vi "UHR-Fleezers Control (fpga) - 11.5.vi"() -> ()   [LabVIEW 2012]
doc: "UHR-Fleezers Instrument Control Code (fpga)"
uses:
  <vilib>/Platform/TimedLoop/XDataNode/timing_clust.ctl
  <vilib>/Platform/TimedLoop/XDataNode/nitl_modes.ctl
  <vilib>/Platform/TimedLoop/XDataNode/wakeup.ctl
  <vilib>/rvi/eio/common/nirviEmuTemplateMethod_errors.vi
  <vilib>/rvi/Emulation/niFpgaSctlEmulationGetInTimedLoop.vi
  <vilib>/rvi/DataTransferAndStorage/Container/Common/niFpgaContainerGetUniqueNameForEmu.vi
  <vilib>/rvi/FIFO/Fifo_Resource/nirvififoEmulationSetSize.vi
  <vilib>/rvi/Emulation/niFpgaSctlEmulationFifoFullMgr.vi
  <vilib>/rvi/errors/niFpgaSetErrorForExecOnDevCompSimple.vi
  <vilib>/rvi/eio/common/nirviEmuReportErrorAndStop.vi
  <vilib>/rvi/interface/RandomDataEmulation/nirviRandomDataFPGAFIFO.vi
  <vilib>/rvi/interface/RandomDataEmulation/niFpgaRandomDataHandleErrors.vi
  <vilib>/rvi/Emulation/niFpgaSctlEmulationGlobalWrite.vi
  <vilib>/rvi/Emulation/niFpgaSctlEmulationRegisterWithScheduler.vi
  <vilib>/rvi/Emulation/niFpgaSctlEmulationScheduler.vi
  <vilib>/rvi/DataTransferAndStorage/Container/Common/niFpgaContainerExecOnDevCompGetState.vi
  <vilib>/rvi/Memory/Memory_Emulation/niFpgaMemoryEmulationCacheClearOnFirstRun.vi
  <vilib>/rvi/Memory/Memory_Emulation/nirvimemoryEmulationManagerCache_MakeExclusive.vi
  <vilib>/rvi/Memory/Memory_Emulation/niFpgaMemoryEmulationValidateCache.vi
  <vilib>/rvi/Memory/Memory_Emulation/nirvimemoryEmulationManagerCache_ReleaseExclusive.vi
  <vilib>/rvi/Memory/Memory_Emulation/nirvimemoryEmulationManagerCache_InsertValue.vi
  <vilib>/Utility/error.llb/Clear Errors.vi
  <vilib>/rvi/Memory/Memory_Emulation/nirvimemoryEmulationManagerCache_GetValue.vi
  <vilib>/rvi/Memory/Memory_Emulation/nirvimemoryEmulationManagerCache_SetValue.vi
  <vilib>/rvi/Emulation/niFpgaSctlEmulationResourceMgr.vi
  <vilib>/Platform/TimedLoop/XDataNode/XDataNode.xnode
  <vilib>/eio/EIOMethodNode/EIOMethodNode.xnode
  <vilib>/eio/EIONode/EIONode.xnode
  <vilib>/rvi/DataTransferAndStorage/Container/XNode/niFpgaContainer.xnode
  <vilib>/rvi/FIFO/Fifo_Resource/nirvififoEmulationRead.vi
  <vilib>/rvi/interface/RandomDataEmulation/nirviRandomDataFpgaReadWriteTemplate.vi
  <vilib>/rvi/Memory/Memory_Emulation/niFpgaMemoryEmulationRefIn.vi
  <vilib>/rvi/FIFO/Fifo_Resource/nirvififoEmulationWrite.vi
  <vilib>/addons/control/pid/fpga.llb/XNode/niFpgaPID.xnode
  <vilib>/Platform/TimedLoop/XDataNode/XDNodeRunTimeDep.lvlib
panel:
  in  "Tab Control":T1(tab)=enum."Force FB"
  in  "Set 3":bool
  in  "Set 2":bool=TRUE
  in  "Set 1":bool=TRUE
  in  "Trap Pos to FIFO":bool
  in  "N of AI1 Int Acq Sets":i16=2 min=1 max=3 step=1
  out "AI Late Counter":u8
  in  "ai count":u16=400
  in  "+ phase":bool
  in  "Phase count adjustment":i16
  out "Relative phase":i16
  in  "AI to FIFO":bool
  out "BD1 Frequency Out 1":u64
  out "BD1 Frequency Out 2":u64
  out "Trap Pos FIFO Timeout":u16
  out "Trap AI FIFO Timeout":u16
  in  "Trap FIFO Set Timeout":i32
  in  "Tab Control 2":T2(tab)
  in  "RD":bool
  in  "FB1 output high":i16=3000
  in  "FB1 output low":i16
  in  "D1":i16
  in  "I1":i16=5
  in  "P1":i16=10
  in  "Swap F1 and F2":bool
  in  "Cont. Scan":bool
  in  "Abort scan":bool
  in  "Cycles per step":u64
  in  "Scan BD":bool
  in  "Number of scans":u16
  in  "Scan steps":u64
  in  "Scan freq.  increment":i64
  out "Scanning":bool
  in  "Start scan":bool
  in  "OSK Bd 1":bool
  in  "Reset Bd 1":bool
  in  "PMODE":bool
  in  "Direct RF Box \nCommunication":bool
  in  "Data BD 2":u8 format="%08b"
  in  "Data BD 1":u8 format="%08b"
  in  "Address":u8 format="%02x"
  in  "Update Data":bool
  in  "FPGA Controls\n RF Box":bool
  in  "Number Interlace Cycles":u8=2 min=1 max=3
  in  "Interlace Off Parameters":u8=1 min=1 max=3
  in  "Interlace ON/OFF":bool
  out "DIO Relative phase":i16
  in  "Phase count adjustment (DIO)":i16
  in  "+ phase (DIO)":bool
  out "DIO Late Counter":u8
  in  "DIO count 1 (ticks)":u16=400
  in  "DIO count 2 (ticks)":u16=400
  in  "DIO count 3 (ticks)":u16=400
  out "AI2 Y Sum Set 2":i16
  out "AI2 Y Sum Set 1":i16
  in  "FB Setpoint Set 1":i16 min=0 step=1
  in  "FB Reset Set 1":bool
  in  "FB On/Off Set 1":bool
  in  "FB Reset Set 2":bool
  in  "FB On/Off Set 2":bool
  in  "FB Setpoint Set 2":i16 min=0 step=1
  out "Scan I":u64
  in  "Amp switch delay":u8=5
  in  "XY phase ext loop method":bool
  in  "BD 2 Amplitude 1":u16
  in  "BD 1 Amplitude 1":u16
  in  "BD 2 Frequency 1":u64
  in  "BD 1 Frequency 1":u64
  in  "BD 2 Amplitude 2":u16
  in  "BD 1 Amplitude 2":u16
  in  "BD 2 Frequency 2":u64
  in  "BD 1 Frequency 2":u64
  in  "BD 2 Amplitude 3":u16
  in  "BD 1 Amplitude 3":u16
  in  "BD 2 Frequency 3":u64
  in  "BD 1 Frequency 3":u64
  in  "BD 1 Delay (ticks)":u8
  in  "BD 2 Delay (Ticks)":u8 caption="Count(Ticks)"
  in  "Next trap write delay (ticks)":u8 caption="Count(Ticks)"
  in  "Amp switch delay 2":u8=5
  in  "BD 2 Delay (Ticks) 2":u8 caption="Count(Ticks)"
  in  "BD 1 Delay (ticks) 2":u8
  in  "Trap 1 osc enable":bool
  in  "N trap osc periods":i16
  in  "Trap osc period (pts)":i16
  in  "Osc traps":bool
  in  "Initiate trap osc":bool
  in  "Ready Write":bool
  in  "Data":i64
  in  "Address 2":u32
  in  "Osc trap cont.":bool
  in  "Trap 2 osc enable":bool
  in  "FB2 output high":fxp<+/-,16,1>=0.999969482421875
  in  "FB2 output low":fxp<+/-,16,1>=-1.0
  in  "P2":fxp<+/-,16,8> format="%.11g"
  in  "I2":fxp<+/-,16,8>=10.0 format="%.11g"
  in  "D2":fxp<+/-,16,8> format="%.11g"
  in  "Negate Diff?":bool
  in  "Diff FB Measurement?":bool
  in  "FB Trig Integrate":u32=1
  out "TTrig?":bool
  in  "TTrig Negate Pos":bool=TRUE
  out "Trap Pos FB Int Signal":fxp<+/-,24,9> format="%.18g"
  out "Trap Pos FB Int-Norm Signal":fxp<+/-,16,1> format="%.16g"
  in  "FPGA TTrig Thresh":i64
  in  "FPGA Trap Trig":bool
  out "Trap Pos FB Action":i64
  in  "Trap Pos. FB Offset Factor":i64
  in  "Trap Pos. FB Mult Factor":i64=2
  in  "Trap Pos. FB Reset":bool
  in  "Trap Pos FB Monitor T1 or T2":bool
  in  "AI1 X Scale":u16
  in  "Trap Pos FB Int Count":u16=100
  in  "Trap Pos FB Negate Action":bool
  out "AI1 X Set 2":fxp<+/-,16,1>
  out "AI1 X Set 1":fxp<+/-,16,1>
  in  "Trap Pos. FB SP":fxp<+/-,16,1>
  in  "Force feedback":bool
  out "TTrig Sig":i64
  out "TTrig Fin Thresh":i64
  in  "1D or 2D Scan?":bool
  in  "Abort scan (MCL)":bool
  in  "MCL Scan Axis":bool
  in  "Cont. Scan (MCL)":bool
  out "Scan I (MCL)":u64
  in  "Number of scans (MCL)":u16
  out "Scanning MCL":bool
  in  "Scan steps (MCL)":u64
  in  "Cycles per step (MCL)":u64
  in  "Scan freq.  increment (MCL)":i16
  in  "Start scan (MCL)":bool
  in  "AO2":i16
  in  "AO1":i16
  out "MCL Late Counter":u8
  in  "MCL count":u32=800
  out "MCL Relative Phase":i16
  in  "Phase count adjustment (MCL)":i16
  in  "+ phase (MCL)":bool
  out "APD3 out state":bool
  in  "APD Gate Operating Mode":u8 max=2 step=1
  in  "Invert APD Gate":bool
  in  "APD Gate OFF Count":u16=100
  in  "APD Gate ON Count":u16=300
  out "APD 1 Gate Late Counter":u8
  out "APD 1 Gate Relative Phase":i16
  in  "Phase count adjustment (APD 1 Gate)":i16
  in  "+ phase (APD 1 Gate)":bool
  out "APD 2 Counts 0":u32
  out "APD 2 Counts 1":u32
  out "APD 1 Counts 0":u32
  out "APD 1 Counts 1":u32
  out "APD1 out state":bool
  in  "APD AO scale factor":i16=1
  in  "APD to FIFO":bool
  in  "APD Acq Rate Count":u32=20000000
  out "APD Acq Late Counter":u8
  out "APD Acq Relative Phase":i16
  in  "Phase Count Adjustment (APD Acq)":i16
  in  "+ phase (APD Acq)":bool
  in  "Phase count adjustment (APD 2 Gate)":i16
  out "APD 2 Gate Late Counter":u8
  out "APD 2 Gate Relative Phase":i16
  in  "+ phase (APD 2 Gate)":bool
  out "APD2 out state":bool
  out "APD 3 Counts 0":u32
  out "APD 3 Counts 1":u32
  out "APD 3 Gate Late Counter":u8
  in  "Phase count adjustment (APD 3 Gate)":i16
  out "APD 3 Gate Relative Phase":i16
  in  "+ phase (APD 3 Gate)":bool
  in  "D3":i16
  in  "I3":i16=5
  in  "P3":i16=10
  in  "Green Filter Flipper":bool
  in  "Green FB Count":u16=1200
  out "Green Late Counter":u8
  out "Green FB Relative Phase":i16
  in  "Phase count adjustment (Green FB)":i16=10
  in  "+ phase (Green FB)":bool
  out "Green FB Sum":i16
  in  "Green int current ON count adj":u16=150
  in  "Current Out":u16=30000
  in  "Green FB On/Off":bool
  in  "Green FB Setpoint":i16=250 min=0 step=1
  in  "Green FB Reset":bool
  in  "Operating Mode 2":u8=2 max=2 step=1
  in  "Invert GI 2":bool
  in  "Green interlace OFF count 2":u16=900
  in  "Green interlace ON count 2":u16=300
  out "GI Late Counter 2":u8
  out "GI Relative phase 2":i16
  in  "Phase count adjustment (GI) 2":i16=20
  in  "+ phase (GI) 2":bool
  in  "Green interlace OFF count":u16=100
  out "GI Relative phase":i16
  in  "Phase count adjustment (GI)":i16
  in  "+ phase (GI)":bool
  in  "Green interlace ON count":u16=300
  out "GI Late Counter":u8
  in  "Invert GI":bool
  in  "Operating Mode":u8 max=2 step=1
  in  "+ phase (RI)":bool
  out "RI Relative phase":i16
  out "RI Late Counter":u8
  in  "Red interlace ON count":u16=300
  in  "Red interlace OFF count":u16=100
  in  "Invert RI":bool
  in  "Red Laser Operating Mode":u8 max=2 step=1
  in  "Phase count adjustment (RI)":i16
  out "Red FB Intensity":i16
  in  "RI Current Out":u16=30000
  in  "Red FB On/Off":bool
  in  "D4":i16
  in  "I4":i16=5
  in  "P4":i16=10
  in  "Red FB Setpoint":i16=250 min=0 step=1
  in  "Red FB Reset":bool
  in  "RI Operating Mode 2":u8=2 max=2 step=1
  in  "Invert RI 2":bool
  in  "Phase count adjustment (BI AO)":i16=20
  in  "Blue current ON count adj (AO)":u16=150
  in  "BI Current Out":i16=30000
  in  "Blue FB On/Off":bool
  in  "D5":i16
  in  "I5":i16=5
  in  "P5":i16=10
  in  "Blue FB Setpoint":i16=250 min=0 step=1
  in  "Blue FB Reset":bool
  in  "BI Operating Mode (AO)":u8=2 max=2 step=1
  in  "Invert BI (AO)":bool
  in  "Blue OFF count (AO)":u16=900
  in  "Blue ON count (AO)":u16=300
  out "BI Late Counter (AO)":u8
  out "BI Relative phase (AO)":i16
  in  "+ phase (BI AO)":bool
  in  "Phase count adjustment (BI D)":i16
  in  "Blue Laser Operating Mode (D)":u8 max=2 step=1
  in  "Invert BI (D)":bool
  in  "Blue interlace OFF count (D)":u16=100
  in  "Blue interlace ON count (D)":u16=300
  out "Blue Late Counter (D)":u8
  out "BI Relative phase (D)":i16
  in  "+ phase (BI D)":bool
  out "Blue Intensity":i16
  # "Only one of these can be on\nat a time:"
  # "Raster Scan AOD"
  # "1 (X)"
  # "2 (Y)"
  # "IR Intensity Feedback (RF BD 1)"
  # "FB Gains Set 1"
  # "FB output range 1"
  # "False is usual, True is external loop method"
  # "Parameters if using the external RF switching loop"
  # "Parameters if using the usual internal RF switching method"
  # "FB Triggering Excitation Laser"
  # "Trap Pos. FB Gains"
  # "Trap Pos. FB Range"
  # "AO1 (Y)"
  # "2D"
  # "1D"
  # "AO2 (X)"
  # "APD AO for aligning"
  # "Detection Loop"
  # "Green fluorescent laser digital gate interlacing loop"
  # "0 Forced ON\n1 Forced OFF\n2 Interlacing"
  # "Green FB Gains"
  # "Red fluorescent laser digital gate interlacing loop"
  # "Detection Loop"
  # "0 Forced ON\n1 Forced OFF\n2 Interlacing"
  # "Analog/FB Control Loop\n(Disabled)"
  # "Digital Control Loop"
  # "Blue laser intensity reading"
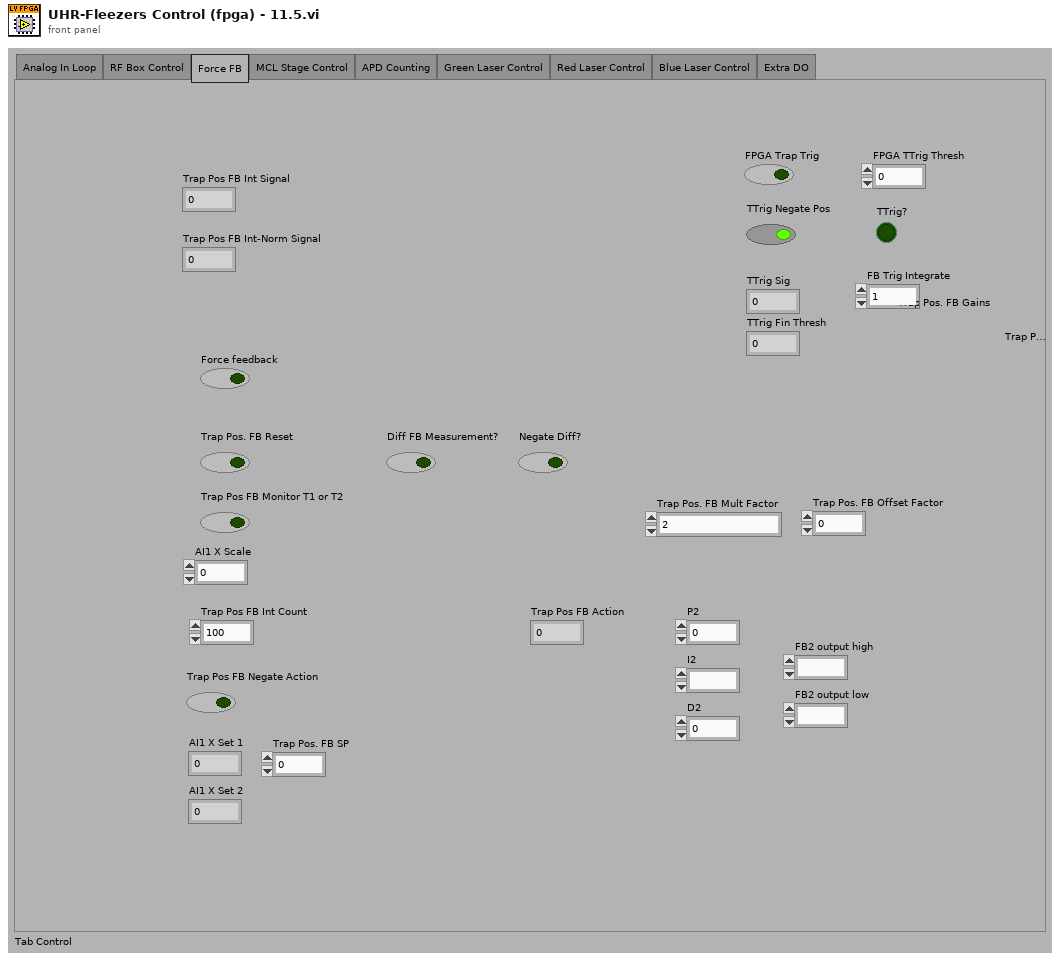
[diagram p1: front panel]
types:
  T1 = enum32{"Analog In Loop", "RF Box Control", "Force FB", "MCL Stage Control", "APD Counting", "Green Laser Control", "Red Laser Control", "Blue Laser Control", "Extra DO"}
  T2 = enum32{"Controls", "Interlacing Frequency and Amplitude Values", "Oscillate trap from memory"}
  T3 = typedef "XDNodeRunTimeDep.lvlib/timing_clust.ctl" = cluster{"Expected End [f-1]":u64, "Actual End [f-1]":u64, "Finished Late? [f-1]":bool, "Expected End [i-1]":u64, "Actual End [i-1]":u64, "Finished Late? [i-1]":bool, "Expected Start [i]":u64, "Actual Start [i]":u64, "Expected Start [f]":u64, "Actual Start [f]":u64, "Source Name":string, "Structure Name":string, "Period":i64, "Deadline":i64, "Offset":i64, "Start":i64, "Priority":i32, "Timeout":i32, "Mode":T4, "Wakeup Reason":T5, "Error":errorcluster, "Source Type":string, "Secondary Source Type":string, "Global End Time":u64, "Global Start Time":u64, "Frame Duration":u64, "Iteration Duration":u64, "Assigned CPU":i32, "I/O Scan Engine Mode":u32}
  T4 = typedef "XDNodeRunTimeDep.lvlib/nitl_modes.ctl" = enum32{"No Change", "Process missed periods, maintain original phase", "Discard missed periods, maintain original phase", "Process missed periods, ignore original phase", "Discard missed periods, ignore original phase"}
  T5 = typedef "XDNodeRunTimeDep.lvlib/wakeup.ctl" = enum32{"Normal", "Aborted", "Asynchronous wakeup", "Timing source error", "Timed loop error", "Timeout"}
  T6 = cluster{"proportional gain (Kc)":i16, "integral gain (Kc*Ts/Ti)":i16, "derivative gain (Kc*Td/Ts)":i16}
  T7 = cluster{"FB1 output high":i16, "FB1 output low":i16}
  T8 = cluster{"P2":fxp<+/-,16,8>, "I2":fxp<+/-,16,8>, "D2":fxp<+/-,16,8>}
  T9 = cluster{"FB2 output high":fxp<+/-,16,1>, "FB2 output low":fxp<+/-,16,1>}
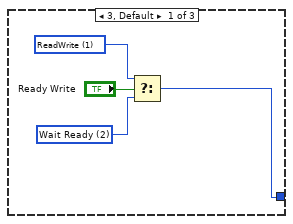
[diagram p2: hidden frame]
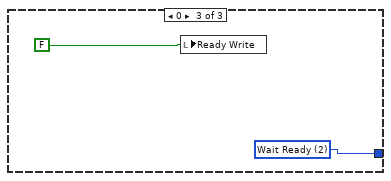
[diagram p3: hidden frame]
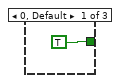
[diagram p5: hidden frame]
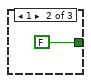
[diagram p6: hidden frame]
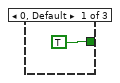
[diagram p7: hidden frame]
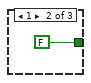
[diagram p8: hidden frame]
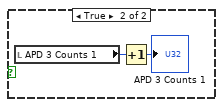
[diagram p9: hidden frame]
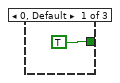
[diagram p10: hidden frame]
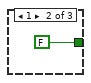
[diagram p11: hidden frame]
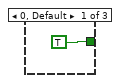
[diagram p12: hidden frame]
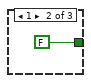
[diagram p13: hidden frame]
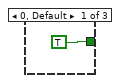
[diagram p14: hidden frame]
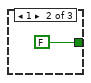
[diagram p15: hidden frame]
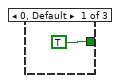
[diagram p16: hidden frame]
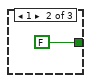
[diagram p17: hidden frame]
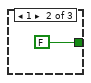
[diagram p20: hidden frame]
diagram:
  w1 = i16 2 items=["UnSet Ready", "ReadWrite", "Wait Ready"]
  w4 = u16 0
  w6 = FALSE
  w3 = FALSE
  # "timing array current index"
  # "timing array"
  # "timing counter (phase adjusted here)"
  # "late counter"
  n1 = while "External XY RF switching timing loop" {
    stop <- FALSE stop-if-true
    # "This loop is stalled until the RF FIFO get a value, which only happens if we are using the external loop RF switching method. With this method we gain additional delay time (because \nwe allow the rest of the main RF loop to procede while this loop waits to send the switch signals - a form of parallelism). Probably this is always the method to use. Helps to simplify \nthe main RF code. If it works reliably, could take out the redundant code in the main RF loop to save space and simplify."
    n2 = xnode ("FIFO Read")("Timeout"=-1) -> ("Element"=w16:bool)  [unwired: 1 in, 2 out]
    n3 = flat-sequence "BD 1 (X)" {
      tunnel: w16 -> [w25]
      tunnel: [w25] -> w15
      tunnel: w15 -> [w27]
      tunnel: "Amp switch delay 2" -> [w28]
      frame #0 {
        n4 = call "Wait9"("Count(Ticks)"="BD 1 Delay (ticks) 2") -> ()  [unwired: 1 out]
      }
      frame #1 {
        # "switch frequency"
        n5 = xnode "FPGA I/O Node"("Connector1/DIO36"=w27) -> ()  [unwired: 1 in, 1 out]
      }
      frame #2 {
        # "~5 ticks is usual"
        n6 = call "Wait10"("Count(Ticks)"=w28) -> ()  [unwired: 1 out]
      }
      frame #3 {
        # "this switches amplitude"
        # "switch amplitude"
        # "send udclk high"
        n7 = xnode "FPGA I/O Node"("Connector1/DIO30"=TRUE ("Connector1/DIO15")) -> ()  [unwired: 1 in, 1 out]
      }
      frame #4 {
        # "reset to be ready for next\ncycle"
        # "send udclk low"
        n8 = xnode "FPGA I/O Node"("Connector1/DIO30"=FALSE ("Connector1/DIO15")) -> ()  [unwired: 1 in, 1 out]
      }
    }
    n9 = flat-sequence "BD 2 (Y)" {
      tunnel: w16 -> [w19]
      tunnel: [w19] -> w14
      tunnel: w14 -> [w21]
      tunnel: "Amp switch delay 2" -> [w22]
      frame #0 {
        n10 = call "Wait11"("Count(Ticks)"="BD 2 Delay (Ticks) 2") -> ()  [unwired: 1 out]
      }
      frame #1 {
        # "switch frequency"
        n11 = xnode "FPGA I/O Node"("Connector1/DIO37"=w21) -> ()  [unwired: 1 in, 1 out]
      }
      frame #2 {
        # "~5 ticks is usual"
        n12 = call "Wait12"("Count(Ticks)"=w22) -> ()  [unwired: 1 out]
      }
      frame #3 {
        # "this switches amplitude"
        # "switch amplitude"
        # "send udclk high"
        n13 = xnode "FPGA I/O Node"("Connector1/DIO29"=TRUE ("Connector1/DIO15")) -> ()  [unwired: 1 in, 1 out]
      }
      frame #4 {
        # "reset to be ready for next\ncycle"
        # "send udclk low"
        n14 = xnode "FPGA I/O Node"("Connector1/DIO29"=FALSE ("Connector1/DIO15")) -> ()  [unwired: 1 in, 1 out]
      }
    }
  }
  n15 = flat-sequence "FPGA initialization to do before running any of the loops" {
    tunnel: [u16 0 ("DIO count 3 (ticks)")] -> w2
    tunnel: [w32] -> _
    frame #0 {
      w31 = FALSE ("Enable")
      # "BD 2 (Y)"
      # "BD 1 (X)"
      # "Start up expansion chassis early\nto avoid delays later"
      # "This pin controls udclk on the RF boards.\nWhen initially configuring the boards, this pin needs to be\nconfigured as a high impedance input.  Later it will be switched\nto an output."
      # "Initial setting of DIO data and \naddress to low (before reset).  \nThis needs to happen before the other\ncontrol method loops execute."
      n16 = xnode "FPGA I/O Node"("Chassis2/Mod4/AO0"=u16 0) -> ("Chassis2/Mod1/AI0"=w32:i16)  [unwired: 2 in, 2 out]
      n17 = xnode "FPGA I/O Method Node"("Enable"=w31) -> ()  [unwired: 1 in, 1 out]
      n18 = xnode "FPGA I/O Method Node"("Enable"=w31) -> ()  [unwired: 1 in, 1 out]
      n19 = xnode "FPGA I/O Node"("Connector1/DIO0"=FALSE, "Connector1/DIO1"=FALSE, "Connector1/DIO2"=FALSE, "Connector1/DIO3"=FALSE, "Connector1/DIO4"=FALSE, "Connector1/DIO5"=FALSE, "Connector1/DIO6"=FALSE, "Connector1/DIO7"=FALSE, "Connector1/DIO8"=FALSE, "Connector1/DIO9"=FALSE, "Connector1/DIO10"=FALSE, "Connector1/DIO11"=FALSE, "Connector1/DIO12"=FALSE, "Connector1/DIO13"=FALSE, "Connector1/DIO15"=FALSE, "Connector1/DIO20"=FALSE, "Connector1/DIO21"=FALSE, "Connector1/DIO22"=FALSE, "Connector1/DIO23"=FALSE, "Connector1/DIO24"=FALSE, "Connector1/DIO25"=FALSE, "Connector1/DIO26"=FALSE, "Connector1/DIO27"=FALSE, "Connector1/DIO14"=FALSE) -> ()  [unwired: 24 in, 24 out]
    }
  }
  n20 = local read "AO1"() -> (w11:i16)
  n21 = local read "AO2"() -> (w10:i16)
  n22 = node-c288() -> (w9:T3)  [unwired: 1 in]
  n23 = timed-loop "RF box board DIO control: control bits" {
    timing: w9 -> [_]
    timing-out: [_] -> w8
    tunnel: [w61] -> _
    tunnel: w2 -> [w61]
    stop <- FALSE stop-if-true
    n24 = xnode "FPGA I/O Node"("Connector1/DIO16"="RD", "Connector1/DIO17"="PMODE", "Connector1/DIO18"="OSK Bd 1", "Connector1/DIO19"="Reset Bd 1", "Connector0/DIO3"="Green Filter Flipper") -> ()  [unwired: 5 in, 5 out]
  }
  n25 = while "Handshake memory transfer for trap oscillation sin wave data" {
    shift-right: [w69] -> _
    shift-left: w1 -> [w70]
    stop <- FALSE stop-if-true
    # "Write"
    n26 = case shown="1" w70 {
      tunnel: [w73 w78 w79] -> w69
      frame 3, Default {
        w71 = i16 2 items=["UnSet Ready", "ReadWrite", "Wait Ready"]
        w72 = i16 1 items=["UnSet Ready", "ReadWrite", "Wait Ready"]
        n27 = Select(t=w72, s="Ready Write", f=w71) -> (s? t:f=w73:i16)
      }
      frame 1 {
        w78 = i16 0 items=["UnSet Ready", "ReadWrite", "Wait Ready"]
        n28 = xnode ("Memory Write")("Address"="Address 2", "Data"="Data", "Memory In"=refnum<k21> "Trap osc memory") -> ()  [unwired: 1 out]
      }
      frame 0 {
        w79 = i16 2 items=["UnSet Ready", "ReadWrite", "Wait Ready"]
        n29 = local write "Ready Write"(FALSE ("Ready Read")) -> ()
      }
    }
  }
  n30 = while "RF box board DIO control: parallel communication" {
    shift-right: [w87] -> _
    shift-left: w2 -> [w86]
    shift-right: [w85] -> _
    shift-left: FALSE ("Swap F1 and F2") -> [w84]
    stop <- FALSE stop-if-true
    n31 = flat-sequence {
      tunnel: w84 -> [w91]
      tunnel: w86 -> [w89]
      tunnel: [w91] -> w83
      tunnel: [w90] -> w82
      tunnel: [w89] -> w81
      tunnel: [w97] -> w87
      tunnel: [w96] -> w85
      tunnel: w83 -> [w95]
      tunnel: w82 -> [w93]
      tunnel: w81 -> [w92]
      frame #0 {
        n32 = call "Loop Timer"("Count(Ticks)"=w89) -> ("Tick Count(Ticks)"=w90:u16)
      }
      frame #1 {
        n33 = flat-sequence {
          tunnel: ["FPGA Controls\n RF Box"] -> w94
          tunnel: w95 -> [w98]
          tunnel: [w156] -> w97
          tunnel: [w169] -> w96
          tunnel: w94 -> [w168]
          tunnel: w93 -> [w162]
          tunnel: w92 -> [w159]
          frame #0 {
            n34 = case shown="True" "FPGA Controls\n RF Box" {
              tunnel: w98 -> [_ w100]
              frame False {
              }
              frame True {
                n35 = flat-sequence {
                  tunnel: w100 -> [w110]
                  frame #0 {
                    n36 = First Call?() -> (First Call?: T/F=w101:bool)
                    n37 = case shown="True" w101 {
                      frame False {
                      }
                      frame True {
                        # "BD 2"
                        # "BD 1"
                        # "If first time data updated, be sure to set WR high and UDCLK low\nbefore setting data and address bits."
                        n38 = xnode "FPGA I/O Method Node"("Enable"=TRUE) -> ("FPGA I/O Out"=w103:refnum<k21>)  [unwired: 1 in]
                        n39 = xnode "FPGA I/O Method Node"("Enable"=TRUE) -> ("FPGA I/O Out"=w106:refnum<k21>)  [unwired: 1 in]
                        n40 = xnode "FPGA I/O Node"("Connector1/DIO15"=TRUE) -> ()  [unwired: 1 in, 1 out]
                        n41 = xnode "FPGA I/O Node"("I/O Item"=FALSE ("Connector1/DIO30"), "FPGA I/O In"=w103) -> ()  [unwired: 1 out]
                        n42 = xnode "FPGA I/O Node"("I/O Item"=FALSE ("Connector1/DIO30"), "FPGA I/O In"=w106) -> ()  [unwired: 1 out]
                      }
                    }
                  }
                  frame #1 {
                    n43 = case shown="True" "XY phase ext loop method" {
                      tunnel: w110 -> [w112 w124]
                      frame False {
                        # "Usual operation"
                        n44 = flat-sequence "BD 1 (X)" {
                          tunnel: w112 -> [w119]
                          tunnel: "Amp switch delay" -> [w120]
                          frame #0 {
                            n45 = call "Wait6"("Count(Ticks)"="BD 1 Delay (ticks)") -> ()  [unwired: 1 out]
                          }
                          frame #1 {
                            # "switch frequency"
                            n46 = xnode "FPGA I/O Node"("Connector1/DIO36"=w119) -> ()  [unwired: 1 in, 1 out]
                          }
                          frame #2 {
                            # "~5 ticks is usual"
                            n47 = call "Wait4"("Count(Ticks)"=w120) -> ()  [unwired: 1 out]
                          }
                          frame #3 {
                            # "this switches amplitude"
                            # "switch amplitude"
                            # "send udclk high"
                            n48 = xnode "FPGA I/O Node"("Connector1/DIO30"=TRUE ("Connector1/DIO15")) -> ()  [unwired: 1 in, 1 out]
                          }
                          frame #4 {
                            # "reset to be ready for next\ncycle"
                            # "send udclk low"
                            n49 = xnode "FPGA I/O Node"("Connector1/DIO30"=FALSE ("Connector1/DIO15")) -> ()  [unwired: 1 in, 1 out]
                          }
                        }
                        n50 = flat-sequence "BD 2 (Y)" {
                          tunnel: w112 -> [w114]
                          tunnel: "Amp switch delay" -> [w115]
                          frame #0 {
                            n51 = call "Wait7"("Count(Ticks)"="BD 2 Delay (Ticks)") -> ()  [unwired: 1 out]
                          }
                          frame #1 {
                            # "switch frequency"
                            n52 = xnode "FPGA I/O Node"("Connector1/DIO37"=w114) -> ()  [unwired: 1 in, 1 out]
                          }
                          frame #2 {
                            # "~5 ticks is usual"
                            n53 = call "Wait5"("Count(Ticks)"=w115) -> ()  [unwired: 1 out]
                          }
                          frame #3 {
                            # "this switches amplitude"
                            # "switch amplitude"
                            # "send udclk high"
                            n54 = xnode "FPGA I/O Node"("Connector1/DIO29"=TRUE ("Connector1/DIO15")) -> ()  [unwired: 1 in, 1 out]
                          }
                          frame #4 {
                            # "reset to be ready for next\ncycle"
                            # "send udclk low"
                            n55 = xnode "FPGA I/O Node"("Connector1/DIO29"=FALSE ("Connector1/DIO15")) -> ()  [unwired: 1 in, 1 out]
                          }
                        }
                      }
                      frame True {
                        # "Operation when you need a long delay for either X or Y to synchonize AOD light out phase (> ~100 ticks)."
                        # "Trigger the external loop by sending the boolean FSK value through a FIFO"
                        n56 = xnode ("FIFO Write")("Element"=w124, "Timeout"=-1) -> ()  [unwired: 1 in, 2 out]
                      }
                    }
                  }
                }
              }
            }
          }
          frame #1 {
            # "This is the prior cycle's on time"
            # "increment timing\nindex, reset to 0 if \nend of matrix"
            # "Reset to begginning (1) when number of cycles reached."
            # "timing index"
            # "build byte stacks for writing data\n(must correspond to addresses array constant)"
            # "Timing housekeeping"
            # "Adjust phase if late\n(maintains constant phase relationship between cycles)"
            n57 = Bundle("FB1 output high"="FB1 output high", "FB1 output low"="FB1 output low") -> (w129:T7)  [unwired: 1 in]
            n58 = Bundle("P1"="P1", "I1"="I1", "D1"="D1") -> (w130:cluster{"P1":i16, "I1":i16, "D1":i16})  [unwired: 1 in]
            n59 = feedback #1(u8 0 ("t")) -> (w165:u8)
            n60 = Increment(x=w165) -> (x+1=w208:u8)
            n61 = Increment(x="Number Interlace Cycles") -> (x+1=w203:u8)
            n62 = Equal?(x=w208, y=w203) -> (x = y?=w210:bool)
            n63 = Select(t=u8 1, s=w210, f=w208) -> (s? t:f=w164:u8)
            n64 = feedback-in #1(w164) -> ()
            n65 = Increment(x=w164) -> (x+1=w205:u8)
            n66 = Equal?(x=w205, y=w203) -> (x = y?=w206:bool)
            n67 = Select(t=u8 1, s=w206, f=w205) -> (s? t:f=w202:u8)
            n68 = Select(t=w202, s="Interlace ON/OFF", f="Interlace Off Parameters") -> (s? t:f=w128:u8)
            n69 = feedback-in #2(w162) -> ()
            n70 = feedback #2(w162) -> (w161:u16)
            n71 = Select(t=w164, s="Interlace ON/OFF", f="Interlace Off Parameters") -> (s? t:f=w201:u8)
            n72 = Subtract(x=w162, y=w161) -> (x-y=w160:u16)
            n73 = Subtract "The error"(x=w160, y=w159) -> (x-y=w137:u16)
            n74 = case shown="1, Default" w201 {
              tunnel: ["DIO count 1 (ticks)" "DIO count 2 (ticks)" "DIO count 3 (ticks)"] -> w158
              frame 1, Default {
              }
              frame 2 {
              }
              frame 3 {
              }
            }
            n75 = Number To Boolean Array(number=w137) -> (Boolean array=w138:bool[])
            n76 = Or Array Elements(Boolean array=w138) -> (logical OR=w136:bool)
            n77 = Boolean To (0,1)(Boolean=w136) -> (0, 1=w143:i16)
            n78 = To Unsigned Byte Integer(number=w143) -> (unsigned 8bit integer=w140:u8)
            n79 = feedback #3(u8 0) -> (w141:u8)
            n80 = Add(x=w140, y=w141) -> (x+y=w139:u8)
            "DIO Late Counter" <- w139
            n81 = feedback-in #3(w139) -> ()
            n82 = Subtract(x=w158, y=w137) -> (x-y=w157:u16)
            n83 = feedback #4(i64 0 ("y")) -> (w126:i64)
            n84 = case "Synchronize trap oscillations - always begin/end with trap 1" shown="1, Default" w128 {
              tunnel: [w211 w212 w213] -> w127
              tunnel: w126 -> [w211 w212 _]
              frame 2 {
              }
              frame 3 {
              }
              frame 1, Default {
                n85 = Or(x="Osc traps", y="Initiate trap osc") -> (x .or. y?=w215:bool)
                n86 = case "Trap sine oscillation (or whatever pattern is stored in memory)" shown="True" w215 {
                  tunnel: [i64 0 ("y") w219] -> w213
                  tunnel: "Initiate trap osc" -> [_ w222]
                  frame False {
                  }
                  frame True {
                    w226 = u16 0
                    w224 = -1
                    n87 = local write "Initiate trap osc"(FALSE ("Initiate trap osc")) -> ()
                    n88 = feedback #5(w226) -> (w228:u16)
                    n89 = Select(t=w226, s=w222, f=w228) -> (s? t:f=w227:u16)
                    n90 = Greater Or Equal?(x=w227, y="Trap osc period (pts)") -> (x >= y?=w233:bool)
                    n91 = Or(x=w222, y=w233) -> (x .or. y?=w234:bool)
                    n92 = Select(t=u16 0, s=w234, f=w227) -> (s? t:f=w218:u16)
                    n93 = feedback #6(w224) -> (w225:i32)
                    n94 = Select(t=w224, s=w222, f=w225) -> (s? t:f=w223:i32)
                    n95 = Increment(x=w223) -> (x+1=w230:i32)
                    n96 = Equal?(x=w218, y=u16 0) -> (x = y?=w231:bool)
                    n97 = Increment(x=w218) -> (x+1=w238:u16)
                    n98 = feedback-in #5(w238) -> ()
                    n99 = Select(t=w230, s=w231, f=w223) -> (s? t:f=w229:i32)
                    n100 = feedback-in #6(w229) -> ()
                    n101 = case shown="False" "Osc trap cont." {
                      tunnel: w229 -> [w242 _]
                      frame False {
                        n102 = Greater Or Equal?(x=w242, y="N trap osc periods") -> (x >= y?=w240:bool)
                        n103 = Not(x=w240) -> (.not. x?=w239:bool)
                        n104 = local write "Osc traps"(w239) -> ()
                      }
                      frame True {
                      }
                    }
                    n105 = xnode "Memory Write"("Address"=w218, "Memory In"=refnum<k21> "Trap osc memory") -> ("Data"=w219:i64)  [unwired: 1 out]
                  }
                }
              }
            }
            n106 = case shown="1, Default" w128 {
              tunnel: [w323 w478 "BD 1 Frequency 3"] -> w198
              tunnel: [w322 "BD 2 Frequency 2" "BD 2 Frequency 3"] -> w187
              tunnel: ["BD 2 Amplitude 1" "BD 2 Amplitude 2" "BD 2 Amplitude 3"] -> w144
              tunnel: [w311 w487 "BD 1 Amplitude 3"] -> w147
              tunnel: w130 -> [w285 w484 _]
              tunnel: w129 -> [w286 w483 _]
              tunnel: w127 -> [w283 w481 _]
              frame 1, Default {
                w302 = fxp<+/-,24,9> 0.0 ("AI1 X Set 2")
                w295 = u16 0
                w318 = u64 0 ("f")
                # "This signal integration happens no matter what\nso that correct setpoints can be chosen before \nturning on the FB."
                # "Trap 1"
                n107 = local read "AI1 X Set 2"() -> (w298:fxp<+/-,16,1>)
                n108 = local read "AI1 X Set 1"() -> (w299:fxp<+/-,16,1>)
                n109 = local read "Scanning"() -> (w324:bool)
                n110 = Or(x=w324, y="Start scan") -> (x .or. y?=w316:bool)
                n111 = case shown="False" "Diff FB Measurement?" {
                  tunnel: w298 -> [w332 w341]
                  tunnel: w299 -> [w331 w342]
                  tunnel: [w329 w333] -> w300
                  frame False {
                    n112 = Select(t=w331, s="Trap Pos FB Monitor T1 or T2", f=w332) -> (s? t:f=w329:fxp<+/-,16,1>)
                  }
                  frame True {
                    n113 = Subtract(x=w342, y=w341) -> (x-y=w334:fxp<+/-,17,2>)
                    n114 = Not(x="Negate Diff?") -> (.not. x?=w340:bool)
                    n115 = Boolean To (0,1)(Boolean="Negate Diff?") -> (0, 1=w338:i16)
                    n116 = Boolean To (0,1)(Boolean=w340) -> (0, 1=w339:i16)
                    n117 = Negate(x=w338) -> (-x=w337:i16)
                    n118 = Add(x=w337, y=w339) -> (x+y=w335:i16)
                    n119 = Multiply(x=w335, y=w334) -> (x*y=w333:fxp<+/-,32,17>)
                  }
                }
                n120 = Not(x="Abort scan") -> (.not. x?=w314:bool)
                n121 = And(x=w314, y=w316) -> (x .and. y?=w313:bool)
                n122 = case "For raster scanning" shown="True" w313 {
                  tunnel: [u64 0 w468] -> w319
                  tunnel: "Start scan" -> [_ w453]
                  frame False {
                    n123 = local write "Scanning"(FALSE ("scanning")) -> ()
                  }
                  frame True {
                    w437 = i64 0
                    w436 = u64 0
                    # "scan incr."
                    # "freq. incr. mult."
                    # "count steps"
                    # "count number of cycles"
                    n124 = feedback #7(w436) -> (w465:u64)
                    n125 = Select(t=w436, s=w453, f=w465) -> (s? t:f=w467:u64)
                    n126 = Increment(x=w467) -> (x+1=w464:u64)
                    n127 = Greater?(x="Cycles per step", y=w464) -> (0:w446:bool)
                    n128 = Select(t=w464, s=w446, f=w436) -> (s? t:f=w463:u64)
                    n129 = feedback-in #7(w463) -> ()
                    n130 = feedback #8(w436) -> (w462:u64)
                    n131 = Select(t=w436, s=w453, f=w462) -> (s? t:f=w457:u64)
                    n132 = Increment(x=w457) -> (x+1=w461:u64)
                    n133 = Add(x="Scan steps", y="Scan steps") -> (x+y=w460:u64)
                    n134 = Select(t=w457, s=w446, f=w461) -> (s? t:f=w441:u64)
                    n135 = Greater?(x=w460, y=w441) -> (0:w440:bool)
                    n136 = Select(t=w441, s=w440, f=w436) -> (s? t:f=w458:u64)
                    n137 = feedback-in #8(w458) -> ()
                    n138 = Equal?(x="Scan steps", y=w441) -> (x = y?=w445:bool)
                    n139 = Greater?(x="Scan steps", y=w457) -> (0:w456:bool)
                    n140 = feedback #9(w437) -> (w459:i64)
                    n141 = Select(t=w437, s=w453, f=w459) -> (s? t:f=w443:i64)
                    n142 = Increment(x=w443) -> (x+1=w455:i64)
                    n143 = Decrement(x=w443) -> (x-1=w454:i64)
                    n144 = Select(t=w455, s=w456, f=w454) -> (s? t:f=w444:i64)
                    n145 = Select(t=w443, s=w445, f=w444) -> (s? t:f=w442:i64)
                    n146 = Select(t=w443, s=w446, f=w442) -> (s? t:f=w438:i64)
                    n147 = Select(t=w438, s=w440, f=w437) -> (s? t:f=w439:i64)
                    n148 = feedback-in #9(w439) -> ()
                    n149 = feedback #10(w436) -> (w452:u64)
                    n150 = Select(t=w436, s=w453, f=w452) -> (s? t:f=w448:u64)
                    n151 = Increment(x=w448) -> (x+1=w449:u64)
                    n152 = Select(t=w448, s=w440, f=w449) -> (s? t:f=w447:u64)
                    n153 = Greater?(x="Number of scans", y=w447) -> (0:w433:bool)
                    n154 = Multiply(x="Scan freq.  increment", y=w443) -> (x*y=w468:i64)
                    n155 = Select(t=TRUE, s="Cont. Scan", f=w433) -> (s? t:f=w432:bool)
                    "Scanning" <- w432
                    n156 = Select(t=w447, s=w432, f=w436) -> (s? t:f=w450:u64)
                    n157 = feedback-in #10(w450) -> ()
                    n158 = Increment(x=w447) -> (x+1=→"Scan I":u64)
                  }
                }
                n159 = feedback #11(w295) -> (w294:u16)
                n160 = Increment(x=w294) -> (x+1=w296:u16)
                n161 = Greater Or Equal?(x=w296, y="Trap Pos FB Int Count") -> (x >= y?=w287:bool)
                n162 = Select(t=w295, s=w287, f=w296) -> (s? t:f=w297:u16)
                n163 = feedback-in #11(w297) -> ()
                n164 = feedback #12(w302) -> (w301:fxp<+/-,24,9>)
                n165 = Add(x=w300, y=w301) -> (x+y=w293:fxp<+/-,24,9>)
                n166 = case "For intensity feedback" shown="True" "FB On/Off Set 1" {
                  tunnel: "BD 1 Amplitude 1" -> [w470 _]
                  tunnel: [w470 w474] -> w311
                  tunnel: w286 -> [_ w471]
                  tunnel: w285 -> [_ w472]
                  frame False {
                  }
                  frame True {
                    n167 = local read "AI2 Y Sum Set 1"() -> (w475:i16)
                    n168 = call "Slower PID.vi"("process variable"=w475, "reset?"="FB Reset Set 1", "setpoint"="FB Setpoint Set 1", "PID gains (x 2^8)"=w472, "output range"=w471) -> ("output"=w476:i16)  [unwired: 10 out]
                    n169 = To Unsigned Word Integer(number=w476) -> (unsigned 16bit integer=w474:u16)
                  }
                }
                n170 = Select(t=w302, s=w287, f=w293) -> (s? t:f=w305:fxp<+/-,24,9>)
                n171 = feedback-in #12(w305) -> ()
                n172 = Divide(x=w293, y="Trap Pos FB Int Count") -> (x/y=w288:fxp<+/-,16,1>)
                n173 = feedback #13(fxp<+/-,24,9> 0.0 ("AI1 X Set 2")) -> (w306:fxp<+/-,24,9>)
                n174 = Select(t=w293, s=w287, f=w306) -> (s? t:f=w307:fxp<+/-,24,9>)
                "Trap Pos FB Int Signal" <- w307
                n175 = feedback-in #13(w307) -> ()
                n176 = feedback #14(fxp<+/-,16,1> 0.0 ("Trap Pos FB Int-Norm Signal")) -> (w290:fxp<+/-,16,1>)
                n177 = Select(t=w288, s=w287, f=w290) -> (s? t:f=w289:fxp<+/-,16,1>)
                "Trap Pos FB Int-Norm Signal" <- w289
                n178 = feedback-in #14(w289) -> ()
                n179 = case "For position feedback" shown="True" "Force feedback" {
                  tunnel: [i64 0 w348] -> w308
                  tunnel: w288 -> [_ w345]
                  tunnel: w287 -> [_ w344]
                  frame False {
                  }
                  frame True {
                    n180 = feedback #15(i64 0) -> (w347:i64)
                    n181 = case shown="True" w344 {
                      tunnel: [w349 w363] -> w348
                      tunnel: w347 -> [w349 _]
                      tunnel: w345 -> [_ w357]
                      frame False {
                      }
                      frame True {
                        w367 = u32 0
                        n182 = Bundle("P2"="P2", "I2"="I2", "D2"="D2") -> (w353:T8)  [unwired: 1 in]
                        n183 = Bundle("FB2 output high"="FB2 output high", "FB2 output low"="FB2 output low") -> (w350:T9)  [unwired: 1 in]
                        n184 = xnode ("PID")("process variable"=w357, "reset?"="Trap Pos. FB Reset", "setpoint"="Trap Pos. FB SP", "PID gains"=w353, "output range"=w350) -> ("output"=w379:fxp<+/-,16,1>)
                        n185 = Negate(x=w379) -> (-x=w378:fxp<+/-,17,2>)
                        n186 = Select(t=w378, s="Trap Pos FB Negate Action", f=w379) -> (s? t:f=w375:fxp<+/-,17,2>)
                        n187 = Scale By Power Of 2(n=u32 15, x=u32 1) -> (x*2^n=w372:u32)
                        n188 = Multiply(x=w375, y=w372) -> (x*y=w371:fxp<+/-,17,17>)
                        n189 = To Quad Integer(1:w371) -> (0:w383:i64)
                        "Trap Pos FB Action" <- w383
                        n190 = Multiply(x=w383, y="Trap Pos. FB Mult Factor") -> (x*y=w381:i64)
                        n191 = Add(x=w381, y="Trap Pos. FB Offset Factor") -> (x+y=w363:i64)
                        n192 = feedback #16() -> (w364:i64)  [unwired: 1 in]
                        n193 = Add(x=w363, y=w364) -> (x+y=w361:i64)
                        n194 = feedback #17(w367) -> (w369:u32)
                        n195 = Increment(x=w369) -> (x+1=w358:u32)
                        n196 = Greater Or Equal?(x=w358, y="FB Trig Integrate") -> (x >= y?=w359:bool)
                        n197 = Select(t=i64 0, s=w359, f=w361) -> (s? t:f=w365:i64)
                        n198 = feedback-in #16(w365) -> ()
                        n199 = Select(t=w367, s=w359, f=w358) -> (s? t:f=w368:u32)
                        n200 = feedback-in #17(w368) -> ()
                        n201 = And(x=w359, y="FPGA Trap Trig") -> (x .and. y?=w366:bool)
                        n202 = case "Trap FB trigger excitation laser ON" shown="True" w366 {
                          tunnel: w361 -> [_ w387]
                          tunnel: w358 -> [_ w385]
                          frame False {
                          }
                          frame True {
                            n203 = Not(x="TTrig Negate Pos") -> (.not. x?=w394:bool)
                            n204 = Boolean To (0,1)(Boolean="TTrig Negate Pos") -> (0, 1=w392:i16)
                            n205 = Boolean To (0,1)(Boolean=w394) -> (0, 1=w393:i16)
                            n206 = Negate(x=w392) -> (-x=w391:i16)
                            n207 = Add(x=w391, y=w393) -> (x+y=w390:i16)
                            n208 = Multiply(x=w390, y=w387) -> (x*y=w389:i64)
                            "TTrig Sig" <- w389
                            n209 = Multiply(x="FPGA TTrig Thresh", y=w385) -> (x*y=w386:i64)
                            "TTrig Fin Thresh" <- w386
                            n210 = Greater Or Equal?(x=w389, y=w386) -> (x >= y?=w388:bool)
                            n211 = case shown="True" w388 {
                              frame False {
                              }
                              frame True {
                                w397 = TRUE ("Green FB On/Off")
                                w399 = u8 2 ("Operating Mode")
                                n212 = local write "Operating Mode 2"(w399) -> ()
                                n213 = local write "Operating Mode"(w399) -> ()
                                n214 = local write "Green FB On/Off"(w397) -> ()
                                n215 = local write "FPGA Trap Trig"(FALSE ("FPGA Trap Trig")) -> ()
                                "TTrig?" <- w397
                              }
                            }
                          }
                        }
                      }
                    }
                    n216 = feedback-in #15(w348) -> ()
                  }
                }
                n217 = Select(t=w283, s="Trap 1 osc enable", f=i64 0) -> (s? t:f=w281:i64)
                n218 = Select(t=w318, s="Scan BD", f=w319) -> (s? t:f=w317:u64)
                n219 = Select(t=w319, s="Scan BD", f=w318) -> (s? t:f=w320:u64)
                n220 = Add(x=w317, y="BD 2 Frequency 1") -> (x+y=w322:u64)
                n221 = Compound Arithmetic op=ADD(w281, "BD 1 Frequency 1", w308, w320) -> (w323:u64)
                "BD1 Frequency Out 1" <- w323
              }
              frame 2 {
                # "Trap 2"
                n222 = case shown="True" "FB On/Off Set 2" {
                  tunnel: [w491 w494] -> w487
                  tunnel: "BD 1 Amplitude 2" -> [w491 _]
                  tunnel: w484 -> [_ w493]
                  tunnel: w483 -> [_ w492]
                  frame False {
                  }
                  frame True {
                    n223 = local read "AI2 Y Sum Set 2"() -> (w497:i16)
                    n224 = call "Slower PID.vi"("process variable"=w497, "reset?"="FB Reset Set 2", "setpoint"="FB Setpoint Set 2", "PID gains (x 2^8)"=w493, "output range"=w492) -> ("output"=w495:i16)  [unwired: 10 out]
                    n225 = To Unsigned Word Integer(number=w495) -> (unsigned 16bit integer=w494:u16)
                  }
                }
                n226 = Select(t=w481, s="Trap 2 osc enable", f=i64 0) -> (s? t:f=w480:i64)
                n227 = Add(x="BD 1 Frequency 2", y=w480) -> (x+y=w478:u64)
                "BD1 Frequency Out 2" <- w478
              }
              frame 3 {
                # "Fluorescence period"
              }
            }
            n228 = feedback-in #4(w127) -> ()
            n229 = Split Number(x=w198) -> (hi(x)=w197:u32, lo(x)=w196:u32)
            n230 = Split Number(x=w187) -> (hi(x)=w192:u32, lo(x)=w191:u32)
            n231 = Boolean To (0,1)(Boolean="+ phase (DIO)") -> (0, 1=w154:i16)
            n232 = Split Number(x=w197) -> (lo(x)=w195:u16)  [unwired: 1 out]
            n233 = Split Number(x=w196) -> (hi(x)=w194:u16, lo(x)=w193:u16)
            n234 = Split Number(x=w192) -> (lo(x)=w190:u16)  [unwired: 1 out]
            n235 = Split Number(x=w191) -> (hi(x)=w189:u16, lo(x)=w188:u16)
            n236 = Split Number(x=w147) -> (hi(x)=w149:u8, lo(x)=w148:u8)
            n237 = Split Number(x=w144) -> (hi(x)=w146:u8, lo(x)=w145:u8)
            n238 = Split Number(x=w195) -> (hi(x)=w186:u8, lo(x)=w185:u8)
            n239 = Split Number(x=w194) -> (hi(x)=w184:u8, lo(x)=w183:u8)
            n240 = Split Number(x=w190) -> (hi(x)=w179:u8, lo(x)=w178:u8)
            n241 = Split Number(x=w193) -> (hi(x)=w182:u8, lo(x)=w181:u8)
            n242 = Split Number(x=w189) -> (hi(x)=w177:u8, lo(x)=w176:u8)
            n243 = Split Number(x=w188) -> (hi(x)=w175:u8, lo(x)=w174:u8)
            n244 = Multiply(x=w154, y="Phase count adjustment (DIO)") -> (x*y=w150:i16)
            n245 = feedback #18(i16 0) -> (w152:i16)
            n246 = Subtract(x=w152, y=w150) -> (x-y=w151:i16)
            "DIO Relative phase" <- w151
            n247 = feedback-in #18(w151) -> ()
            n248 = Add(x=w157, y=w150) -> (x+y=w156:u16)
            n249 = Build Array "BD 1 A Stack"(w149, w148) -> (w171:u8[])
            n250 = Build Array "BD 2 A Stack"(w146, w145) -> (w170:u8[])
            n251 = Build Array "BD 1 nu Stack"(w186, w185, w184, w183, w182, w181) -> (w180:u8[])
            n252 = Build Array "BD 2 nu Stack"(w179, w178, w177, w176, w175, w174) -> (w173:u8[])
            n253 = case shown="2" w128 {
              tunnel: [w273 w276] -> w169
              tunnel: [u8 10 u8 4] -> w172
              tunnel: "Swap F1 and F2" -> [w274 w276]
              frame 2 {
                # "F2"
                n254 = Not(x=w274) -> (.not. x?=w273:bool)
              }
              frame 1, Default {
                # "low chooses F1"
                # "F1"
              }
            }
            n255 = case "If FPGA is controlling (toggling) RF synth" shown="True" w168 {
              tunnel: w180 -> [_ w249]
              tunnel: w173 -> [_ w248]
              tunnel: w172 -> [_ w247]
              tunnel: w171 -> [_ w246]
              tunnel: w170 -> [_ w245]
              frame False {
              }
              frame True {
                # "Write next amp.\n(wait until beginning of next loop iteration to update)"
                n256 = flat-sequence "Update the next F1 and F2 frequency value (the actual frequency won't change until FSK is switched).\nThen load the next amplitude value into buffer, but don't update it until the next cycle." {
                  tunnel: w248 -> [w251]
                  tunnel: w249 -> [w252]
                  tunnel: [w252] -> w244
                  tunnel: [w251] -> w243
                  tunnel: w247 -> [w253]
                  tunnel: w244 -> [w255]
                  tunnel: w243 -> [w254]
                  tunnel: w246 -> [w266]
                  tunnel: w245 -> [w265]
                  frame #0 {
                    # "To possibly send\nthese writes to very\nend of loop (for x and\ny phase adjust)"
                    n257 = call "Wait8"("Count(Ticks)"="Next trap write delay (ticks)") -> ()  [unwired: 1 out]
                  }
                  frame #1 {
                    n258 = for {
                      tunnel: w255 -> [w261] mode=indexing
                      tunnel: w254 -> [w260] mode=indexing
                      tunnel: w253 -> [w258]
                      i -> [w259]
                      # "Write next freq."
                      n259 = To Unsigned Byte Integer(number=w259) -> (unsigned 8bit integer=w256:u8)
                      n260 = Add(x=w258, y=w256) -> (x+y=w257:u8)
                      n261 = call "write to RF synth bd.vi"("Address Byte"=w257, "BD 2 Byte"=w260, "BD 1 Byte"=w261) -> ()
                    }
                  }
                  frame #2 {
                    w262 = TRUE ("Connector1/DIO15")
                    # "send udclk high\n(BD 1 and 2)"
                    n262 = xnode "FPGA I/O Node"("Connector1/DIO30"=w262, "Connector1/DIO29"=w262) -> ()  [unwired: 2 in, 2 out]
                  }
                  frame #3 {
                    w263 = FALSE ("Connector1/DIO15")
                    n263 = xnode "FPGA I/O Node"("Connector1/DIO30"=w263, "Connector1/DIO29"=w263) -> ()  [unwired: 2 in, 2 out]
                  }
                  frame #4 {
                    n264 = for {
                      tunnel: w266 -> [w272] mode=indexing
                      tunnel: w265 -> [w271] mode=indexing
                      tunnel: u8 33 -> [w269]
                      i -> [w270]
                      n265 = To Unsigned Byte Integer(number=w270) -> (unsigned 8bit integer=w267:u8)
                      n266 = Add(x=w269, y=w267) -> (x+y=w268:u8)
                      n267 = call "write to RF synth bd.vi"("Address Byte"=w268, "BD 2 Byte"=w271, "BD 1 Byte"=w272) -> ()
                    }
                  }
                }
              }
            }
          }
        }
      }
    }
  }
  n268 = while "RF box board direct communication loop" {
    tunnel: w2 -> [_]
    stop <- FALSE stop-if-true
    n269 = case "Whether to use direct communication method (only use one method at a time)" shown="True" "Direct RF Box \nCommunication" {
      frame False {
      }
      frame True {
        n270 = case shown="True" "Update Data" {
          frame False {
          }
          frame True {
            n271 = flat-sequence {
              frame #0 {
                n272 = First Call?() -> (First Call?: T/F=w506:bool)
                n273 = case shown="True" w506 {
                  frame False {
                  }
                  frame True {
                    # "If first time data updated, be sure to set WR high\nbefore setting data and address bits."
                    n274 = flat-sequence {
                      frame #0 {
                        n275 = xnode "FPGA I/O Node"("Connector1/DIO15"=TRUE) -> ()  [unwired: 1 in, 1 out]
                      }
                      frame #1 {
                        n276 = call "Wait"("Count(Ticks)"=u8 40 ("DO Delay 3 (Ticks)")) -> ()  [unwired: 1 out]
                      }
                    }
                  }
                }
              }
              frame #1 {
                n277 = Number To Boolean Array(number="Address") -> (Boolean array=w555:bool[])
                n278 = Number To Boolean Array(number="Data BD 1") -> (Boolean array=w556:bool[])
                n279 = Number To Boolean Array(number="Data BD 2") -> (Boolean array=w525:bool[])
                n280 = Index Array(array=w556, index=7) -> (element=w540:bool)
                n281 = Index Array(array=w556, index=6) -> (element=w539:bool)
                n282 = Index Array(array=w556, index=5) -> (element=w538:bool)
                n283 = Index Array(array=w556, index=4) -> (element=w537:bool)
                n284 = Index Array(array=w556, index=3) -> (element=w536:bool)
                n285 = Index Array(array=w556, index=2) -> (element=w535:bool)
                n286 = Index Array(array=w556, index=1) -> (element=w534:bool)
                n287 = Index Array(array=w556, index=0) -> (element=w533:bool)
                n288 = Index Array(array=w555, index=5) -> (element=w532:bool)
                n289 = Index Array(array=w555, index=4) -> (element=w531:bool)
                n290 = Index Array(array=w555, index=3) -> (element=w530:bool)
                n291 = Index Array(array=w555, index=2) -> (element=w529:bool)
                n292 = Index Array(array=w555, index=1) -> (element=w528:bool)
                n293 = Index Array(array=w555, index=0) -> (element=w527:bool)
                n294 = Index Array(array=w525, index=7) -> (element=w516:bool)
                n295 = Index Array(array=w525, index=6) -> (element=w515:bool)
                n296 = Index Array(array=w525, index=5) -> (element=w514:bool)
                n297 = Index Array(array=w525, index=4) -> (element=w513:bool)
                n298 = Index Array(array=w525, index=3) -> (element=w512:bool)
                n299 = Index Array(array=w525, index=2) -> (element=w511:bool)
                n300 = Index Array(array=w525, index=1) -> (element=w510:bool)
                n301 = Index Array(array=w525, index=0) -> (element=w509:bool)
                n302 = xnode "FPGA I/O Node"("Connector1/DIO0"=w540, "Connector1/DIO1"=w539, "Connector1/DIO2"=w538, "Connector1/DIO3"=w537, "Connector1/DIO4"=w536, "Connector1/DIO5"=w535, "Connector1/DIO6"=w534, "Connector1/DIO7"=w533, "Connector1/DIO8"=w532, "Connector1/DIO9"=w531, "Connector1/DIO10"=w530, "Connector1/DIO11"=w529, "Connector1/DIO12"=w528, "Connector1/DIO13"=w527, "Connector1/DIO20"=w516, "Connector1/DIO21"=w515, "Connector1/DIO22"=w514, "Connector1/DIO23"=w513, "Connector1/DIO24"=w512, "Connector1/DIO25"=w511, "Connector1/DIO26"=w510, "Connector1/DIO27"=w509) -> ()  [unwired: 22 in, 22 out]
              }
              frame #2 {
                # "wait and then apply write signal"
                n303 = call "Wait2"("Count(Ticks)"=u8 40 ("DO Delay 1 (Ticks)")) -> ()  [unwired: 1 out]
              }
              frame #3 {
                # "sending bit low writes data to board buffer"
                n304 = xnode "FPGA I/O Node"("Connector1/DIO15"=FALSE) -> ()  [unwired: 1 in, 1 out]
              }
              frame #4 {
                # "wait then return write signal"
                n305 = call "Wait3"("Count(Ticks)"=u8 40 ("DO Delay 2 (Ticks)")) -> ()  [unwired: 1 out]
              }
              frame #5 {
                # "sending bit high makes ready to\nwrite more data"
                n306 = xnode "FPGA I/O Node"("Connector1/DIO15"=TRUE) -> ()  [unwired: 1 in, 1 out]
              }
            }
          }
        }
      }
    }
  }
  n307 = To Unsigned Long Integer(number=w2) -> (unsigned 32bit integer=w7:u32)
  n308 = while "APD 1 Counter" {
    tunnel: w2 -> [_]
    stop <- FALSE stop-if-true
    n309 = flat-sequence {
      frame #0 {
        n310 = xnode "FPGA I/O Method Node"("FPGA I/O In"=refnum<k21> "Connector0/DIO0" ("APD 1 DO"), "Timeout"=-1) -> ()  [unwired: 2 out]
      }
      frame #1 {
        n311 = local read "APD1 out state"() -> (w566:bool)
        n312 = case shown="False" w566 {
          frame False {
            n313 = local read "APD 1 Counts 0"() -> (w568:u32)
            n314 = Increment(x=w568) -> (x+1=→"APD 1 Counts 0":u32)
          }
          frame True {
            n315 = local read "APD 1 Counts 1"() -> (w570:u32)
            n316 = Increment(x=w570) -> (x+1=→"APD 1 Counts 1":u32)
          }
        }
      }
    }
  }
  n317 = while "APD 2 Counter" {
    tunnel: w2 -> [_]
    stop <- FALSE stop-if-true
    n318 = flat-sequence {
      frame #0 {
        n319 = xnode "FPGA I/O Method Node"("FPGA I/O In"=refnum<k21> "Connector0/DIO1" ("APD 2 DO"), "Timeout"=-1) -> ()  [unwired: 2 out]
      }
      frame #1 {
        n320 = local read "APD2 out state"() -> (w574:bool)
        n321 = case shown="False" w574 {
          frame False {
            n322 = local read "APD 2 Counts 0"() -> (w576:u32)
            n323 = Increment(x=w576) -> (x+1=→"APD 2 Counts 0":u32)
          }
          frame True {
            n324 = local read "APD 2 Counts 1"() -> (w578:u32)
            n325 = Increment(x=w578) -> (x+1=→"APD 2 Counts 1":u32)
          }
        }
      }
    }
  }
  n326 = while "APD 2 Gating" {
    shift-right: [w582] -> _
    shift-left: w2 -> [w587]
    shift-right: [w581] -> _
    shift-left: w6 -> [w579]
    stop <- FALSE stop-if-true
    n327 = flat-sequence {
      tunnel: w587 -> [w590]
      tunnel: [w591] -> w585
      tunnel: [w590] -> w583
      tunnel: [w589] -> w580
      tunnel: w579 -> [w589]
      tunnel: [w594] -> w586
      tunnel: w585 -> [w594]
      tunnel: [w593] -> w584
      tunnel: w583 -> [w593]
      tunnel: w580 -> [w592]
      tunnel: [w612] -> w582
      tunnel: w586 -> [w623]
      tunnel: w584 -> [w621]
      tunnel: [w616] -> w581
      frame #0 {
        n328 = call "Loop Timer8"("Count(Ticks)"=w590) -> ("Tick Count(Ticks)"=w591:u16)
      }
      frame #1 {
        # "Signal is then sent through \na transistor before APD"
        n329 = xnode "FPGA I/O Node"("Connector0/DIO8"=w592) -> ()  [unwired: 1 in, 1 out]
      }
      frame #2 {
        n330 = local read "APD Gate ON Count"() -> (w605:u16)
        n331 = local read "APD Gate OFF Count"() -> (w604:u16)
        n332 = feedback #19(TRUE) -> (w618:bool)
        n333 = feedback-in #20(w623) -> ()
        n334 = feedback #20(w623) -> (w606:u16)
        n335 = Not(x=w618) -> (.not. x?=w615:bool)
        n336 = feedback-in #19(w615) -> ()
        n337 = Subtract(x=w623, y=w606) -> (x-y=w622:u16)
        n338 = Select(t=w605, s=w615, f=w604) -> (s? t:f=w620:u16)
        n339 = Subtract(x=w622, y=w621) -> (x-y=w597:u16)
        n340 = Subtract(x=w620, y=w597) -> (x-y=w611:u16)
        n341 = Number To Boolean Array(number=w597) -> (Boolean array=w596:bool[])
        n342 = Or Array Elements(Boolean array=w596) -> (logical OR=w595:bool)
        n343 = Boolean To (0,1)(Boolean="+ phase (APD 2 Gate)") -> (0, 1=w609:i16)
        n344 = Multiply(x=w609, y="Phase count adjustment (APD 2 Gate)") -> (x*y=w607:i16)
        n345 = Boolean To (0,1)(Boolean=w595) -> (0, 1=w602:i16)
        n346 = Add(x=w611, y=w607) -> (x+y=w612:u16)
        n347 = To Unsigned Byte Integer(number=w602) -> (unsigned 8bit integer=w599:u8)
        n348 = feedback #21(i16 0) -> (w614:i16)
        n349 = Subtract(x=w614, y=w607) -> (x-y=w613:i16)
        "APD 2 Gate Relative Phase" <- w613
        n350 = feedback-in #21(w613) -> ()
        n351 = feedback #22(u8 0) -> (w600:u8)
        n352 = Add(x=w599, y=w600) -> (x+y=w598:u8)
        "APD 2 Gate Late Counter" <- w598
        n353 = feedback-in #22(w598) -> ()
        n354 = local read "APD Gate Operating Mode"() -> (w603:u8)
        n355 = case shown="2" w603 {
          tunnel: [TRUE FALSE w629] -> w616
          tunnel: w618 -> [_ _ w627]
          frame 0, Default {
          }
          frame 1 {
          }
          frame 2 {
            n356 = local read "Invert APD Gate"() -> (w626:bool)
            n357 = Not(x=w627) -> (.not. x?=w628:bool)
            n358 = Select(t=w628, s=w626, f=w627) -> (s? t:f=w629:bool)
          }
        }
      }
    }
  }
  n359 = while "532 nm green fluorescent laser interlacing (DO to IA 532 nm AOM ME amp)." {
    shift-right: [w633] -> _
    shift-left: w2 -> [w638]
    shift-right: [w632] -> _
    shift-left: w3 -> [w630]
    stop <- FALSE stop-if-true
    n360 = flat-sequence {
      tunnel: w638 -> [w641]
      tunnel: [w642] -> w636
      tunnel: [w641] -> w634
      tunnel: [w640] -> w631
      tunnel: w630 -> [w640]
      tunnel: [w645] -> w637
      tunnel: w636 -> [w645]
      tunnel: [w644] -> w635
      tunnel: w634 -> [w644]
      tunnel: w631 -> [w643]
      tunnel: [w654] -> w633
      tunnel: w637 -> [w674]
      tunnel: w635 -> [w671]
      tunnel: [w663] -> w632
      frame #0 {
        n361 = call "Loop Timer4"("Count(Ticks)"=w641) -> ("Tick Count(Ticks)"=w642:u16)
      }
      frame #1 {
        # "Then to PRL 440 amp"
        n362 = xnode "FPGA I/O Node"("Connector1/DIO39"=w643) -> ()  [unwired: 1 in, 1 out]
      }
      frame #2 {
        n363 = feedback-in #23(w674) -> ()
        n364 = feedback #23(w674) -> (w673:u16)
        n365 = Subtract(x=w674, y=w673) -> (x-y=w672:u16)
        n366 = Subtract(x=w672, y=w671) -> (x-y=w647:u16)
        n367 = Number To Boolean Array(number=w647) -> (Boolean array=w648:bool[])
        n368 = Or Array Elements(Boolean array=w648) -> (logical OR=w646:bool)
        n369 = Boolean To (0,1)(Boolean="+ phase (GI)") -> (0, 1=w659:i16)
        n370 = Multiply(x=w659, y="Phase count adjustment (GI)") -> (x*y=w656:i16)
        n371 = Boolean To (0,1)(Boolean=w646) -> (0, 1=w653:i16)
        n372 = To Unsigned Byte Integer(number=w653) -> (unsigned 8bit integer=w650:u8)
        n373 = feedback #24(i16 0) -> (w657:i16)
        n374 = feedback #25(u8 0) -> (w651:u8)
        n375 = Add(x=w650, y=w651) -> (x+y=w649:u8)
        "GI Late Counter" <- w649
        n376 = feedback-in #25(w649) -> ()
        n377 = Subtract(x=w657, y=w656) -> (x-y=w655:i16)
        "GI Relative phase" <- w655
        n378 = feedback-in #24(w655) -> ()
        n379 = feedback #26(TRUE) -> (w666:bool)
        n380 = case shown="2" "Operating Mode" {
          tunnel: [TRUE FALSE w680] -> w663
          tunnel: w666 -> [_ _ w677]
          frame 0, Default {
          }
          frame 1 {
          }
          frame 2 {
            n381 = Not(x=w677) -> (.not. x?=w679:bool)
            n382 = Select(t=w679, s="Invert GI", f=w677) -> (s? t:f=w680:bool)
          }
        }
        n383 = Not(x=w666) -> (.not. x?=w662:bool)
        n384 = Select(t="Green interlace ON count", s=w662, f="Green interlace OFF count") -> (s? t:f=w668:u16)
        n385 = Subtract(x=w668, y=w647) -> (x-y=w660:u16)
        n386 = Add(x=w660, y=w656) -> (x+y=w654:u16)
        n387 = feedback-in #26(w662) -> ()
      }
    }
  }
  n388 = while "Green and red fluorescent laser interlacing (Current AO to IA 532 nm AOM ME amp)." {
    shift-right: [w689] -> _
    shift-left: w2 -> [w692]
    shift-right: [w686] -> _
    shift-left: w4 -> [w684]
    shift-right: [w683] -> _
    shift-left: w4 -> [w682]
    stop <- FALSE stop-if-true
    n389 = flat-sequence {
      tunnel: w692 -> [w696]
      tunnel: [w697] -> w691
      tunnel: [w696] -> w690
      tunnel: [w695] -> w685
      tunnel: w684 -> [w695]
      tunnel: w682 -> [w694]
      tunnel: [w694] -> w681
      tunnel: [w701] -> w688
      tunnel: w691 -> [w701]
      tunnel: [w700] -> w687
      tunnel: w690 -> [w700]
      tunnel: w685 -> [w699]
      tunnel: w681 -> [w698]
      tunnel: [w722] -> w689
      tunnel: [w738] -> w686
      tunnel: w688 -> [w749]
      tunnel: w687 -> [w746]
      tunnel: [w706] -> w683
      frame #0 {
        n390 = call "Loop Timer10"("Count(Ticks)"=w696) -> ("Tick Count(Ticks)"=w697:u16)
      }
      frame #1 {
        n391 = xnode "FPGA I/O Node"("Chassis2/Mod4/AO0"=w699, "Chassis2/Mod4/AO1"=w698) -> ()  [unwired: 2 in, 2 out]
      }
      frame #2 {
        # "Design note:\n\nThese two laser controls are in the same loop\nbecause the expansion current AI cannot separately\ntime the outputs fast enough for us.  Apparently\nit is because of communication time between the\nexpansion card and the fpga.\n\nSo the two analog control signals have the same timing\nand profile, but independent amplitudes to independently\ncontrol the intensity and feedback for each laser."
        n392 = feedback #27(TRUE) -> (w702:bool)
        n393 = Not(x=w702) -> (.not. x?=w703:bool)
        n394 = feedback-in #27(w703) -> ()
        n395 = Subtract(x="Green interlace OFF count 2", y="Green int current ON count adj") -> (x-y=w731:u16)
        n396 = feedback-in #28(w749) -> ()
        n397 = feedback #28(w749) -> (w748:u16)
        n398 = Add(x="Green int current ON count adj", y="Green interlace ON count 2") -> (x+y=w732:u16)
        n399 = Subtract(x=w749, y=w748) -> (x-y=w747:u16)
        n400 = Select(t=w732, s=w703, f=w731) -> (s? t:f=w743:u16)
        n401 = Subtract(x=w747, y=w746) -> (x-y=w715:u16)
        n402 = case shown="2" "RI Operating Mode 2" {
          tunnel: [TRUE FALSE w755] -> w704
          tunnel: w702 -> [_ _ w752]
          frame 0, Default {
          }
          frame 1 {
          }
          frame 2 {
            n403 = Not(x=w752) -> (.not. x?=w754:bool)
            n404 = Select(t=w754, s="Invert RI 2", f=w752) -> (s? t:f=w755:bool)
          }
        }
        n405 = Subtract(x=w743, y=w715) -> (x-y=w726:u16)
        n406 = case shown="0, Default" "Operating Mode 2" {
          tunnel: [TRUE FALSE w789] -> w707
          tunnel: w702 -> [_ _ w786]
          frame 0, Default {
          }
          frame 1 {
          }
          frame 2 {
            n407 = Not(x=w786) -> (.not. x?=w788:bool)
            n408 = Select(t=w788, s="Invert GI 2", f=w786) -> (s? t:f=w789:bool)
          }
        }
        n409 = Number To Boolean Array(number=w715) -> (Boolean array=w716:bool[])
        n410 = Boolean To (0,1)(Boolean="+ phase (GI) 2") -> (0, 1=w728:i16)
        n411 = Or Array Elements(Boolean array=w716) -> (logical OR=w714:bool)
        n412 = Boolean To (0,1)(Boolean=w714) -> (0, 1=w721:i16)
        n413 = Multiply(x=w728, y="Phase count adjustment (GI) 2") -> (x*y=w724:i16)
        n414 = To Unsigned Byte Integer(number=w721) -> (unsigned 8bit integer=w717:u8)
        n415 = Add(x=w726, y=w724) -> (x+y=w722:u16)
        n416 = feedback #29(u8 0) -> (w719:u8)
        n417 = Add(x=w717, y=w719) -> (x+y=w718:u8)
        "GI Late Counter 2" <- w718
        n418 = feedback-in #29(w718) -> ()
        n419 = feedback #30(i16 0) -> (w725:i16)
        n420 = Subtract(x=w725, y=w724) -> (x-y=w723:i16)
        "GI Relative phase 2" <- w723
        n421 = feedback-in #30(w723) -> ()
        n422 = And(x=w707, y="Green FB On/Off") -> (x .and. y?=w733:bool)
        n423 = And(x=w704, y="Red FB On/Off") -> (x .and. y?=w713:bool)
        n424 = case shown="True" w733 {
          tunnel: "Current Out" -> [w770 _]
          tunnel: [w770 w779] -> w737
          frame False {
          }
          frame True {
            n425 = local read "Green FB Sum"() -> (w775:i16)
            n426 = Bundle("P3"="P3", "I3"="I3", "D3"="D3") -> (w771:cluster{"P3":i16, "I3":i16, "D3":i16})  [unwired: 1 in]
            n427 = call "Slower PID.vi"("process variable"=w775, "reset?"="Green FB Reset", "setpoint"="Green FB Setpoint", "PID gains (x 2^8)"=w771, "output range"=cluster{"output high":i16, "output low":i16} {"output high"=32767, "output low"=-32768} ("Green FB output range")) -> ("output"=w782:i16)  [unwired: 10 out]
            n428 = To Long Integer(number=w782) -> (32bit integer=w776:i32)
            n429 = Add(x=w776, y=32768) -> (x+y=w778:i32)
            n430 = To Unsigned Word Integer(number=w778) -> (unsigned 16bit integer=w779:u16)
          }
        }
        n431 = case shown="True" w713 {
          tunnel: "RI Current Out" -> [w756 _]
          tunnel: [w756 w765] -> w709
          frame False {
          }
          frame True {
            n432 = local read "Red FB Intensity"() -> (w761:i16)
            n433 = Bundle("P4"="P4", "I4"="I4", "D4"="D4") -> (w757:cluster{"P4":i16, "I4":i16, "D4":i16})  [unwired: 1 in]
            n434 = call "Slower PID.vi"("process variable"=w761, "reset?"="Red FB Reset", "setpoint"="Red FB Setpoint", "PID gains (x 2^8)"=w757, "output range"=cluster{"output high":i16, "output low":i16} {"output high"=32767, "output low"=-32768} ("Green FB output range")) -> ("output"=w768:i16)  [unwired: 10 out]
            n435 = To Long Integer(number=w768) -> (32bit integer=w762:i32)
            n436 = Add(x=w762, y=32768) -> (x+y=w764:i32)
            n437 = To Unsigned Word Integer(number=w764) -> (unsigned 16bit integer=w765:u16)
          }
        }
        n438 = Boolean To (0,1)(Boolean=w707) -> (0, 1=w739:i16)
        n439 = Boolean To (0,1)(Boolean=w704) -> (0, 1=w708:i16)
        n440 = To Unsigned Word Integer(number=w739) -> (unsigned 16bit integer=w736:u16)
        n441 = To Unsigned Word Integer(number=w708) -> (unsigned 16bit integer=w710:u16)
        n442 = Multiply(x=w736, y=w737) -> (x*y=w738:u16)
        n443 = Multiply(x=w710, y=w709) -> (x*y=w706:u16)
      }
    }
  }
  n444 = while "MCL stage control" {
    shift-right: [w802] -> _
    shift-left: w2 -> [w805]
    shift-right: [w795] -> _
    shift-left: w11 -> [w792]
    shift-right: [w794] -> _
    shift-left: w10 -> [w790]
    stop <- FALSE stop-if-true
    n445 = flat-sequence {
      tunnel: w805 -> [w809]
      tunnel: [w810] -> w801
      tunnel: [w809] -> w799
      tunnel: [w808] -> w793
      tunnel: w792 -> [w808]
      tunnel: [w807] -> w791
      tunnel: w790 -> [w807]
      tunnel: w801 -> [w814]
      tunnel: [w814] -> w800
      tunnel: w799 -> [w813]
      tunnel: [w813] -> w798
      tunnel: w793 -> [w812]
      tunnel: w791 -> [w811]
      tunnel: w800 -> [w822]
      tunnel: w798 -> [w821]
      tunnel: [w822] -> w804
      tunnel: [w821] -> w803
      tunnel: [w820] -> w797
      tunnel: [w819] -> w796
      tunnel: [w894] -> w802
      tunnel: w804 -> [w901]
      tunnel: w803 -> [w898]
      tunnel: w797 -> [w896]
      tunnel: w796 -> [w895]
      tunnel: [w896] -> w795
      tunnel: [w895] -> w794
      frame #0 {
        n446 = call "Loop Timer5"("Count(Ticks)"=w809) -> ("Tick Count(Ticks)"=w810:u32)
      }
      frame #1 {
        n447 = xnode "FPGA I/O Node"("Connector0/AO1"=w812, "Connector0/AO2"=w811) -> ()  [unwired: 2 in, 2 out]
      }
      frame #2 {
        n448 = local read "Scanning MCL"() -> (w834:bool)
        n449 = Or(x=w834, y="Start scan (MCL)") -> (x .or. y?=w829:bool)
        n450 = Not(x="Abort scan (MCL)") -> (.not. x?=w827:bool)
        n451 = And(x=w827, y=w829) -> (x .and. y?=w826:bool)
        n452 = case "Raster scan" shown="True" w826 {
          tunnel: [w835 w878] -> w831
          tunnel: "Start scan (MCL)" -> [_ w863]
          tunnel: [w835 w839] -> w815
          frame False {
            w835 = i16 0
            n453 = local write "Scanning MCL"(FALSE ("scanning")) -> ()
          }
          frame True {
            w849 = i16 0
            w848 = u64 0
            # "scan incr."
            # "freq. incr. mult."
            # "count steps"
            # "count number of cycles"
            n454 = feedback #31(w848) -> (w875:u64)
            n455 = Select(t=w848, s=w863, f=w875) -> (s? t:f=w877:u64)
            n456 = Increment(x=w877) -> (x+1=w874:u64)
            n457 = Greater?(x="Cycles per step (MCL)", y=w874) -> (0:w858:bool)
            n458 = Select(t=w874, s=w858, f=w848) -> (s? t:f=w873:u64)
            n459 = feedback-in #31(w873) -> ()
            n460 = feedback #32(w848) -> (w872:u64)
            n461 = Select(t=w848, s=w863, f=w872) -> (s? t:f=w867:u64)
            n462 = Increment(x=w867) -> (x+1=w871:u64)
            n463 = Add(x="Scan steps (MCL)", y="Scan steps (MCL)") -> (x+y=w870:u64)
            n464 = Select(t=w867, s=w858, f=w871) -> (s? t:f=w853:u64)
            n465 = Greater?(x=w870, y=w853) -> (0:w852:bool)
            n466 = Select(t=w853, s=w852, f=w848) -> (s? t:f=w868:u64)
            n467 = feedback-in #32(w868) -> ()
            n468 = Equal?(x="Scan steps (MCL)", y=w853) -> (x = y?=w857:bool)
            n469 = Greater?(x="Scan steps (MCL)", y=w867) -> (0:w866:bool)
            n470 = feedback #33(w849) -> (w869:i16)
            n471 = Select(t=w849, s=w863, f=w869) -> (s? t:f=w855:i16)
            n472 = Increment(x=w855) -> (x+1=w865:i16)
            n473 = Decrement(x=w855) -> (x-1=w864:i16)
            n474 = Select(t=w865, s=w866, f=w864) -> (s? t:f=w856:i16)
            n475 = Select(t=w855, s=w857, f=w856) -> (s? t:f=w854:i16)
            n476 = Select(t=w855, s=w858, f=w854) -> (s? t:f=w850:i16)
            n477 = Select(t=w850, s=w852, f=w849) -> (s? t:f=w851:i16)
            n478 = feedback-in #33(w851) -> ()
            n479 = feedback #34(w848) -> (w862:u64)
            n480 = Select(t=w848, s=w863, f=w862) -> (s? t:f=w837:u64)
            n481 = Increment(x=w837) -> (x+1=w859:u64)
            n482 = Select(t=w837, s=w852, f=w859) -> (s? t:f=w838:u64)
            n483 = Greater?(x="Number of scans (MCL)", y=w838) -> (0:w845:bool)
            n484 = Multiply(x="Scan freq.  increment (MCL)", y=w855) -> (x*y=w878:i16)
            n485 = Select(t=TRUE, s="Cont. Scan (MCL)", f=w845) -> (s? t:f=w844:bool)
            "Scanning MCL" <- w844
            n486 = Select(t=w838, s=w844, f=w848) -> (s? t:f=w860:u64)
            n487 = feedback-in #34(w860) -> ()
            n488 = Increment(x=w838) -> (x+1=→"Scan I (MCL)":u64)
            n489 = To Word Integer(number=w837) -> (16bit integer=w840:i16)
            n490 = Multiply(x=w840, y="Scan freq.  increment (MCL)") -> (x*y=w839:i16)
          }
        }
        n491 = Select(t=w815, s="1D or 2D Scan?", f=i16 0) -> (s? t:f=w816:i16)
        n492 = Select(t=w816, s="MCL Scan Axis", f=w831) -> (s? t:f=w830:i16)
        n493 = Select(t=w831, s="MCL Scan Axis", f=w816) -> (s? t:f=w832:i16)
        n494 = Add(x=w830, y="AO2") -> (x+y=w819:i16)
        n495 = Add(x="AO1", y=w832) -> (x+y=w820:i16)
      }
      frame #3 {
        n496 = feedback-in #35(w901) -> ()
        n497 = feedback #35(w901) -> (w900:u32)
        n498 = Boolean To (0,1)(Boolean="+ phase (MCL)") -> (0, 1=w892:i16)
        n499 = Subtract(x=w901, y=w900) -> (x-y=w899:u32)
        n500 = Multiply(x=w892, y="Phase count adjustment (MCL)") -> (x*y=w888:i16)
        n501 = Subtract(x=w899, y=w898) -> (x-y=w880:u32)
        n502 = Subtract(x="MCL count", y=w880) -> (x-y=w890:u32)
        n503 = feedback #36(i16 0) -> (w889:i16)
        n504 = Subtract(x=w889, y=w888) -> (x-y=w887:i16)
        "MCL Relative Phase" <- w887
        n505 = feedback-in #36(w887) -> ()
        n506 = Number To Boolean Array(number=w880) -> (Boolean array=w881:bool[])
        n507 = Or Array Elements(Boolean array=w881) -> (logical OR=w879:bool)
        n508 = Boolean To (0,1)(Boolean=w879) -> (0, 1=w886:i16)
        n509 = Add(x=w890, y=w888) -> (x+y=w894:u32)
        n510 = To Unsigned Byte Integer(number=w886) -> (unsigned 8bit integer=w883:u8)
        n511 = feedback #37(u8 0) -> (w884:u8)
        n512 = Add(x=w883, y=w884) -> (x+y=w882:u8)
        "MCL Late Counter" <- w882
        n513 = feedback-in #37(w882) -> ()
      }
    }
  }
  n514 = while "Excitation laser intensity feedback measurement (all lasers)" {
    shift-right: [w903] -> _
    shift-left: w2 -> [w908]
    stop <- FALSE stop-if-true
    n515 = flat-sequence {
      tunnel: w908 -> [w910]
      tunnel: [w911] -> w906
      tunnel: [w910] -> w904
      tunnel: [w917] -> w907
      tunnel: w906 -> [w917]
      tunnel: [w916] -> w905
      tunnel: w904 -> [w916]
      tunnel: [w929] -> w903
      tunnel: w907 -> [w940]
      tunnel: w905 -> [w937]
      frame #0 {
        n516 = call "Loop Timer9"("Count(Ticks)"=w910) -> ("Tick Count(Ticks)"=w911:u16)
      }
      frame #1 {
        # "Design note:\n\nAll lasers need to be measured at the same \ntime because the AI expansion module\ncannot independently time the measurements\nwithin our requirements: their is dead time.\n\nThis probably wouldn't be an issue with the built\nin AI on the fpga board itself."
        n517 = xnode "FPGA I/O Node"("Connector1/DIO35"=TRUE) -> ("Chassis2/Mod1/AI2"=→"Blue Intensity":i16, "Chassis2/Mod1/AI1"=→"Red FB Intensity":i16, "Chassis2/Mod1/AI0"=→"Green FB Sum":i16)  [unwired: 4 in, 4 out]
      }
      frame #2 {
        n518 = feedback-in #38(w940) -> ()
        n519 = feedback #38(w940) -> (w939:u16)
        n520 = Subtract(x=w940, y=w939) -> (x-y=w938:u16)
        n521 = xnode "FPGA I/O Node"("Connector1/DIO35"=FALSE) -> ()  [unwired: 1 in, 1 out]
        n522 = Subtract(x=w938, y=w937) -> (x-y=w919:u16)
        n523 = Subtract(x="Green FB Count", y=w919) -> (x-y=w933:u16)
        n524 = Number To Boolean Array(number=w919) -> (Boolean array=w920:bool[])
        n525 = Or Array Elements(Boolean array=w920) -> (logical OR=w918:bool)
        n526 = Boolean To (0,1)(Boolean="+ phase (Green FB)") -> (0, 1=w931:i16)
        n527 = Boolean To (0,1)(Boolean=w918) -> (0, 1=w925:i16)
        n528 = Multiply(x=w931, y="Phase count adjustment (Green FB)") -> (x*y=w926:i16)
        n529 = Add(x=w933, y=w926) -> (x+y=w929:u16)
        n530 = To Unsigned Byte Integer(number=w925) -> (unsigned 8bit integer=w922:u8)
        n531 = feedback #39(i16 0) -> (w928:i16)
        n532 = Subtract(x=w928, y=w926) -> (x-y=w927:i16)
        "Green FB Relative Phase" <- w927
        n533 = feedback-in #39(w927) -> ()
        n534 = feedback #40(u8 0) -> (w923:u8)
        n535 = Add(x=w922, y=w923) -> (x+y=w921:u8)
        "Green Late Counter" <- w921
        n536 = feedback-in #40(w921) -> ()
      }
    }
  }
  n537 = while "APD 1 Gating" {
    shift-right: [w944] -> _
    shift-left: w2 -> [w949]
    shift-right: [w943] -> _
    shift-left: w6 -> [w941]
    stop <- FALSE stop-if-true
    n538 = flat-sequence {
      tunnel: w949 -> [w952]
      tunnel: [w953] -> w947
      tunnel: [w952] -> w945
      tunnel: [w951] -> w942
      tunnel: w941 -> [w951]
      tunnel: [w956] -> w948
      tunnel: w947 -> [w956]
      tunnel: [w955] -> w946
      tunnel: w945 -> [w955]
      tunnel: w942 -> [w954]
      tunnel: [w970] -> w944
      tunnel: w948 -> [w985]
      tunnel: w946 -> [w982]
      tunnel: [w974] -> w943
      frame #0 {
        n539 = call "Loop Timer7"("Count(Ticks)"=w952) -> ("Tick Count(Ticks)"=w953:u16)
      }
      frame #1 {
        # "Signal is then sent through \na transistor before APD"
        n540 = xnode "FPGA I/O Node"("Connector0/DIO4"=w954) -> ()  [unwired: 1 in, 1 out]
      }
      frame #2 {
        n541 = feedback #41(TRUE) -> (w977:bool)
        n542 = feedback-in #42(w985) -> ()
        n543 = feedback #42(w985) -> (w984:u16)
        n544 = Not(x=w977) -> (.not. x?=w973:bool)
        n545 = feedback-in #41(w973) -> ()
        n546 = Subtract(x=w985, y=w984) -> (x-y=w983:u16)
        n547 = Select(t="APD Gate ON Count", s=w973, f="APD Gate OFF Count") -> (s? t:f=w979:u16)
        n548 = Subtract(x=w983, y=w982) -> (x-y=w958:u16)
        n549 = Subtract(x=w979, y=w958) -> (x-y=w969:u16)
        n550 = Number To Boolean Array(number=w958) -> (Boolean array=w959:bool[])
        n551 = Or Array Elements(Boolean array=w959) -> (logical OR=w957:bool)
        n552 = Boolean To (0,1)(Boolean="+ phase (APD 1 Gate)") -> (0, 1=w967:i16)
        n553 = Boolean To (0,1)(Boolean=w957) -> (0, 1=w964:i16)
        n554 = Multiply(x=w967, y="Phase count adjustment (APD 1 Gate)") -> (x*y=w965:i16)
        n555 = To Unsigned Byte Integer(number=w964) -> (unsigned 8bit integer=w961:u8)
        n556 = Add(x=w969, y=w965) -> (x+y=w970:u16)
        n557 = feedback #43(i16 0) -> (w972:i16)
        n558 = Subtract(x=w972, y=w965) -> (x-y=w971:i16)
        "APD 1 Gate Relative Phase" <- w971
        n559 = feedback-in #43(w971) -> ()
        n560 = feedback #44(u8 0) -> (w962:u8)
        n561 = Add(x=w961, y=w962) -> (x+y=w960:u8)
        "APD 1 Gate Late Counter" <- w960
        n562 = feedback-in #44(w960) -> ()
        n563 = case shown="2" "APD Gate Operating Mode" {
          tunnel: [TRUE FALSE w991] -> w974
          tunnel: w977 -> [_ _ w988]
          frame 0, Default {
          }
          frame 1 {
          }
          frame 2 {
            n564 = Not(x=w988) -> (.not. x?=w990:bool)
            n565 = Select(t=w990, s="Invert APD Gate", f=w988) -> (s? t:f=w991:bool)
          }
        }
      }
    }
  }
  n566 = while "Control APD data integration - stream to host" {
    shift-right: [w995] -> _
    shift-left: w7 -> [w1000]
    stop <- FALSE stop-if-true
    n567 = flat-sequence {
      tunnel: w1000 -> [w1002]
      tunnel: [w1003] -> w998
      tunnel: [w1002] -> w996
      tunnel: [w1013] -> w999
      tunnel: w998 -> [w1013]
      tunnel: [w1012] -> w997
      tunnel: w996 -> [w1012]
      tunnel: [w1011] -> w994
      tunnel: [w1010] -> w993
      tunnel: [w1004] -> w992
      tunnel: [w1055] -> w995
      tunnel: w999 -> [w1065]
      tunnel: w997 -> [w1062]
      tunnel: w994 -> [w1048]
      tunnel: w993 -> [w1047]
      tunnel: w992 -> [w1035]
      frame #0 {
        n568 = call "Loop Timer6"("Count(Ticks)"=w1002) -> ("Tick Count(Ticks)"=w1003:u32)
      }
      frame #1 {
        n569 = flat-sequence {
          tunnel: [w1015] -> w1009
          tunnel: w1009 -> [w1018]
          tunnel: [w1022] -> w1008
          tunnel: [w1021] -> w1007
          tunnel: [w1018] -> w1006
          tunnel: [w1017] -> w1005
          tunnel: [w1029] -> w1010
          tunnel: [w1030] -> w1011
          tunnel: w1008 -> [w1030]
          tunnel: w1007 -> [w1029]
          tunnel: w1006 -> [w1028]
          tunnel: w1005 -> [w1027]
          tunnel: [w1027] -> w1004
          frame #0 {
            # "use separate variable so each APD won't\nhave to wait to read"
            n570 = feedback #45(FALSE) -> (w1014:bool)
            "APD1 out state" <- w1014
            "APD2 out state" <- w1014
            "APD3 out state" <- w1014
            n571 = Not(x=w1014) -> (.not. x?=w1015:bool)
            n572 = feedback-in #45(w1015) -> ()
          }
          frame #1 {
            n573 = local read "APD 3 Counts 1"() -> (w1020:u32)
            n574 = local read "APD 3 Counts 0"() -> (w1019:u32)
            n575 = local read "APD 1 Counts 1"() -> (w1026:u32)
            n576 = local read "APD 1 Counts 0"() -> (w1025:u32)
            n577 = local read "APD 2 Counts 1"() -> (w1024:u32)
            n578 = local read "APD 2 Counts 0"() -> (w1023:u32)
            n579 = Select(t=w1020, s=w1018, f=w1019) -> (s? t:f=w1017:u32)
            n580 = Select(t=w1026, s=w1018, f=w1025) -> (s? t:f=w1022:u32)
            n581 = Select(t=w1024, s=w1018, f=w1023) -> (s? t:f=w1021:u32)
          }
          frame #2 {
            n582 = case shown="False" w1028 {
              frame False {
                w1031 = u32 0 ("APD 1 Counts 0")
                n583 = local write "APD 1 Counts 0"(w1031) -> ()
                n584 = local write "APD 2 Counts 0"(w1031) -> ()
                n585 = local write "APD 3 Counts 0"(w1031) -> ()
              }
              frame True {
                w1032 = u32 0 ("APD 1 Counts 1")
                n586 = local write "APD 1 Counts 1"(w1032) -> ()
                n587 = local write "APD 2 Counts 1"(w1032) -> ()
                n588 = local write "APD 3 Counts 1"(w1032) -> ()
              }
            }
          }
        }
      }
      frame #2 {
        n589 = feedback-in #46(w1065) -> ()
        n590 = feedback #46(w1065) -> (w1064:u32)
        n591 = Subtract(x=w1065, y=w1064) -> (x-y=w1063:u32)
        n592 = Subtract(x=w1063, y=w1062) -> (x-y=w1040:u32)
        n593 = case shown="True" "APD to FIFO" {
          tunnel: w1048 -> [_ w1070]
          tunnel: w1047 -> [_ w1068]
          tunnel: w1035 -> [_ w1066]
          frame False {
          }
          frame True {
            n594 = flat-sequence {
              tunnel: 0 ("Timeout") -> [w1072]
              tunnel: w1070 -> [w1073]
              tunnel: [w1072] -> w1069
              tunnel: w1069 -> [w1074]
              tunnel: w1068 -> [w1075]
              tunnel: [w1074] -> w1067
              tunnel: w1067 -> [w1077]
              tunnel: w1066 -> [w1076]
              frame #0 {
                n595 = xnode ("FIFO Write")("Element"=w1073, "Timeout"=w1072) -> ()  [unwired: 1 in, 2 out]
              }
              frame #1 {
                n596 = xnode ("FIFO Write")("Element"=w1075, "Timeout"=w1074) -> ()  [unwired: 1 in, 2 out]
              }
              frame #2 {
                n597 = xnode ("FIFO Write")("Element"=w1076, "Timeout"=w1077) -> ()  [unwired: 1 in, 2 out]
              }
            }
          }
        }
        n598 = Subtract(x="APD Acq Rate Count", y=w1040) -> (x-y=w1056:u32)
        n599 = Number To Boolean Array(number=w1040) -> (Boolean array=w1041:bool[])
        n600 = Or Array Elements(Boolean array=w1041) -> (logical OR=w1039:bool)
        n601 = Boolean To (0,1)(Boolean=w1039) -> (0, 1=w1046:i16)
        n602 = To Unsigned Byte Integer(number=w1046) -> (unsigned 8bit integer=w1043:u8)
        n603 = feedback #47(u8 0) -> (w1044:u8)
        n604 = Add(x=w1043, y=w1044) -> (x+y=w1042:u8)
        "APD Acq Late Counter" <- w1042
        n605 = feedback-in #47(w1042) -> ()
        n606 = Boolean To (0,1)(Boolean="+ phase (APD Acq)") -> (0, 1=w1052:i16)
        n607 = Multiply(x=w1052, y="Phase Count Adjustment (APD Acq)") -> (x*y=w1049:i16)
        n608 = Add(x=w1056, y=w1049) -> (x+y=w1055:u32)
        n609 = feedback #48(i16 0) -> (w1054:i16)
        n610 = Subtract(x=w1054, y=w1049) -> (x-y=w1051:i16)
        "APD Acq Relative Phase" <- w1051
        n611 = feedback-in #48(w1051) -> ()
        n612 = To Word Integer(number=w1048) -> (16bit integer=w1057:i16)
        n613 = To Word Integer(number=w1035) -> (16bit integer=w1036:i16)
        n614 = To Word Integer(number=w1047) -> (16bit integer=w1058:i16)
        n615 = Multiply(x="APD AO scale factor", y=w1058) -> (x*y=w1037:i16)
        n616 = Multiply(x="APD AO scale factor", y=w1036) -> (x*y=w1033:i16)
        n617 = Multiply(x="APD AO scale factor", y=w1057) -> (x*y=w1038:i16)
        n618 = xnode "FPGA I/O Node"("Connector0/AO5"=w1038, "Connector0/AO7"=w1037, "Connector0/AO6"=w1033) -> ()  [unwired: 3 in, 3 out]
      }
    }
  }
  n619 = while "DAQ AI set 1" {
    shift-right: [w1078] -> _
    shift-left: w2 -> [w1083]
    stop <- FALSE stop-if-true
    n620 = flat-sequence {
      tunnel: w1083 -> [w1093]
      tunnel: [w1094] -> w1081
      tunnel: [w1093] -> w1080
      tunnel: [w1104] -> w1091
      tunnel: [w1103] -> w1090
      tunnel: [w1102] -> w1089
      tunnel: [w1101] -> w1088
      tunnel: [w1100] -> w1087
      tunnel: [w1099] -> w1086
      tunnel: [w1098] -> w1085
      tunnel: [w1097] -> w1084
      tunnel: [w1096] -> w1082
      tunnel: w1081 -> [w1096]
      tunnel: w1080 -> [w1095]
      tunnel: [w1095] -> w1079
      tunnel: [w1133] -> w1078
      tunnel: w1091 -> [w1160]
      tunnel: w1090 -> [w1125]
      tunnel: w1089 -> [w1126]
      tunnel: w1088 -> [w1159]
      tunnel: w1087 -> [w1149]
      tunnel: w1086 -> [w1148]
      tunnel: w1085 -> [w1147]
      tunnel: w1084 -> [w1146]
      tunnel: w1082 -> [w1143]
      tunnel: w1079 -> [w1140]
      frame #0 {
        n621 = call "Loop Timer3"("Count(Ticks)"=w1093) -> ("Tick Count(Ticks)"=w1094:u16)
      }
      frame #1 {
        n622 = xnode "FPGA I/O Node"("Connector1/DIO31"=TRUE ("Connector1/DIO33")) -> ("Connector0/AI0"=w1104:i16, "Connector0/AI1"=w1103:i16, "Connector0/AI2"=w1102:i16, "Connector0/AI3"=w1101:i16, "Connector0/AI4"=w1100:i16, "Connector0/AI5"=w1099:i16, "Connector0/AI6"=w1098:i16, "Connector0/AI7"=w1097:i16)  [unwired: 9 in, 9 out]
      }
      frame #2 {
        w1129 = FALSE ("AI to FIFO")
        # "Adjust phase after data acquired if button pressed"
        n623 = feedback #49(i16 1) -> (w1152:i16)
        n624 = Increment(x=w1152) -> (x+1=w1158:i16)
        n625 = Scale By Power Of 2(n="AI1 X Scale", x=w1125) -> (x*2^n=w1123:i16)
        n626 = Greater?(x=w1158, y="N of AI1 Int Acq Sets") -> (0:w1155:bool)
        n627 = Select(t=i16 1, s=w1155, f=w1158) -> (s? t:f=w1157:i16)
        n628 = feedback-in #49(w1157) -> ()
        n629 = Divide(x=w1123, y=w1126) -> (x/y=w1122:fxp<+/-,16,1>)
        n630 = feedback #50(w1129) -> (w1127:bool)
        n631 = feedback #51(w1129) -> (w1145:bool)
        n632 = case shown="2" w1152 {
          tunnel: w1126 -> [w1183 w1190 _]
          tunnel: ["Set 1" "Set 2" "Set 3"] -> w1150
          tunnel: ["AI to FIFO" w1192 w1197] -> w1144
          tunnel: w1145 -> [_ w1192 w1197]
          tunnel: ["Trap Pos to FIFO" w1191 w1196] -> w1128
          tunnel: w1127 -> [_ w1191 w1196]
          tunnel: w1122 -> [w1182 w1189 _]
          tunnel: [w1181 w1187 FALSE] -> w1109
          tunnel: [w1180 w1188 u64 0 ("BD1 Frequency Out 2")] -> w1108
          frame 1, Default {
            n633 = local read "BD1 Frequency Out 1"() -> (w1180:u64)
            n634 = Compound Arithmetic op=AND("Trap Pos to FIFO", "Set 1", "AI to FIFO") -> (w1181:bool)
            "AI2 Y Sum Set 1" <- w1183
            "AI1 X Set 1" <- w1182
          }
          frame 2 {
            n635 = local read "BD1 Frequency Out 2"() -> (w1188:u64)
            n636 = Compound Arithmetic op=AND(w1191, "Set 2", w1192) -> (w1187:bool)
            "AI2 Y Sum Set 2" <- w1190
            "AI1 X Set 2" <- w1189
          }
          frame 3 {
          }
        }
        n637 = And(x=w1150, y=w1144) -> (x .and. y?=w1151:bool)
        n638 = case shown="True" w1151 {
          tunnel: w1160 -> [_ w1211]
          tunnel: w1125 -> [_ w1210]
          tunnel: w1126 -> [_ w1209]
          tunnel: w1159 -> [_ w1208]
          tunnel: w1149 -> [_ w1207]
          tunnel: w1148 -> [_ w1206]
          tunnel: w1147 -> [_ w1205]
          tunnel: w1146 -> [_ w1204]
          tunnel: 0 ("DMA buffer timeout") -> [_ w1213]
          frame False {
          }
          frame True {
            n639 = Build Array(w1211, w1210, w1209, w1208, w1207, w1206, w1205, w1204) -> (w1212:i16[])
            n640 = for {
              tunnel: w1212 -> [w1215] mode=indexing
              tunnel: w1213 -> [w1216]
              tunnel: [w1214] -> w1202 mode=indexing
              n641 = xnode ("FIFO Write")("Element"=w1215, "Timeout"=w1216) -> ("Timed Out?"=w1214:bool)  [unwired: 1 in, 1 out]
            }
            n642 = Or Array Elements(Boolean array=w1202) -> (logical OR=w1199:bool)
            n643 = Boolean To (0,1)(Boolean=w1199) -> (0, 1=w1201:i16)
            n644 = feedback #52(u16 0) -> (w1200:u16)
            n645 = Add(x=w1201, y=w1200) -> (x+y=w1198:u16)
            "Trap AI FIFO Timeout" <- w1198
            n646 = feedback-in #52(w1198) -> ()
          }
        }
        n647 = feedback-in #50(w1128) -> ()
        n648 = feedback-in #51(w1144) -> ()
        n649 = case shown="True" w1109 {
          tunnel: w1108 -> [_ w1166]
          tunnel: [u8 0 w1163] -> w1107
          frame False {
          }
          frame True {
            n650 = Split Number(x=w1166) -> (hi(x)=w1167:u32, lo(x)=w1168:u32)
            n651 = Split Number(x=w1167) -> (lo(x)=w1169:u16)  [unwired: 1 out]
            n652 = Split Number(x=w1168) -> (hi(x)=w1170:u16, lo(x)=w1171:u16)
            n653 = Build Array "BD 1 nu Stack"(w1169, w1170, w1171) -> (w1165:u16[])
            n654 = for {
              tunnel: w1165 -> [w1178] mode=indexing
              shift-right: [w1174] -> w1163
              shift-left: u8 0 -> [w1175]
              n655 = xnode ("FIFO Method Node")("Element"=w1178, "Timeout"="Trap FIFO Set Timeout") -> ("Timed Out?"=w1177:bool)  [unwired: 1 in, 1 out]
              n656 = Boolean To (0,1)(Boolean=w1177) -> (0, 1=w1176:i16)
              n657 = To Unsigned Byte Integer(number=w1176) -> (unsigned 8bit integer=w1173:u8)
              n658 = Add(x=w1173, y=w1175) -> (x+y=w1174:u8)
            }
          }
        }
        n659 = To Unsigned Word Integer(number=w1107) -> (unsigned 16bit integer=w1106:u16)
        n660 = feedback #53(u16 0) -> (w1120:u16)
        n661 = Add(x=w1106, y=w1120) -> (x+y=w1119:u16)
        "Trap Pos FIFO Timeout" <- w1119
        n662 = feedback-in #53(w1119) -> ()
        n663 = feedback-in #54(w1143) -> ()
        n664 = feedback #54(w1143) -> (w1142:u16)
        n665 = Subtract(x=w1143, y=w1142) -> (x-y=w1141:u16)
        n666 = xnode "FPGA I/O Node"("Connector1/DIO31"=FALSE ("Connector1/DIO34")) -> ()  [unwired: 1 in, 1 out]
        n667 = Subtract(x=w1141, y=w1140) -> (x-y=w1111:u16)
        n668 = Boolean To (0,1)(Boolean="+ phase") -> (0, 1=w1136:i16)
        n669 = Multiply(x=w1136, y="Phase count adjustment") -> (x*y=w1130:i16)
        n670 = Subtract(x="ai count", y=w1111) -> (x-y=w1134:u16)
        n671 = Number To Boolean Array(number=w1111) -> (Boolean array=w1112:bool[])
        n672 = feedback #55(i16 0) -> (w1132:i16)
        n673 = Add(x=w1134, y=w1130) -> (x+y=w1133:u16)
        n674 = Subtract(x=w1132, y=w1130) -> (x-y=w1131:i16)
        "Relative phase" <- w1131
        n675 = feedback-in #55(w1131) -> ()
        n676 = Or Array Elements(Boolean array=w1112) -> (logical OR=w1110:bool)
        n677 = Boolean To (0,1)(Boolean=w1110) -> (0, 1=w1117:i16)
        n678 = To Unsigned Byte Integer(number=w1117) -> (unsigned 8bit integer=w1114:u8)
        n679 = feedback #56(u8 0) -> (w1115:u8)
        n680 = Add(x=w1114, y=w1115) -> (x+y=w1113:u8)
        "AI Late Counter" <- w1113
        n681 = feedback-in #56(w1113) -> ()
      }
    }
  }
  n682 = node-c288(w8) -> ()
  n683 = while "APD 3 Counter" {
    tunnel: w2 -> [_]
    stop <- FALSE stop-if-true
    n684 = flat-sequence {
      frame #0 {
        n685 = xnode "FPGA I/O Method Node"("FPGA I/O In"=refnum<k21> "Connector0/DIO2" ("APD 2 DO"), "Timeout"=-1) -> ()  [unwired: 2 out]
      }
      frame #1 {
        n686 = local read "APD3 out state"() -> (w1220:bool)
        n687 = case shown="False" w1220 {
          frame False {
            n688 = local read "APD 3 Counts 0"() -> (w1222:u32)
            n689 = Increment(x=w1222) -> (x+1=→"APD 3 Counts 0":u32)
          }
          frame True {
            n690 = local read "APD 3 Counts 1"() -> (w1224:u32)
            n691 = Increment(x=w1224) -> (x+1=→"APD 3 Counts 1":u32)
          }
        }
      }
    }
  }
  n692 = while "APD 3 Gating" {
    shift-right: [w1228] -> _
    shift-left: w2 -> [w1233]
    shift-right: [w1227] -> _
    shift-left: w6 -> [w1225]
    stop <- FALSE stop-if-true
    n693 = flat-sequence {
      tunnel: w1233 -> [w1236]
      tunnel: [w1237] -> w1231
      tunnel: [w1236] -> w1229
      tunnel: [w1235] -> w1226
      tunnel: w1225 -> [w1235]
      tunnel: [w1240] -> w1232
      tunnel: w1231 -> [w1240]
      tunnel: [w1239] -> w1230
      tunnel: w1229 -> [w1239]
      tunnel: w1226 -> [w1238]
      tunnel: [w1257] -> w1228
      tunnel: w1232 -> [w1269]
      tunnel: w1230 -> [w1266]
      tunnel: [w1261] -> w1227
      frame #0 {
        n694 = call "Loop Timer15"("Count(Ticks)"=w1236) -> ("Tick Count(Ticks)"=w1237:u16)
      }
      frame #1 {
        # "Signal is then sent through \na transistor before APD"
        n695 = xnode "FPGA I/O Node"("Connector0/DIO9"=w1238) -> ()  [unwired: 1 in, 1 out]
      }
      frame #2 {
        n696 = local read "APD Gate OFF Count"() -> (w1242:u16)
        n697 = local read "APD Gate ON Count"() -> (w1243:u16)
        n698 = feedback #57(TRUE) -> (w1263:bool)
        n699 = feedback-in #58(w1269) -> ()
        n700 = feedback #58(w1269) -> (w1268:u16)
        n701 = Not(x=w1263) -> (.not. x?=w1260:bool)
        n702 = feedback-in #57(w1260) -> ()
        n703 = Subtract(x=w1269, y=w1268) -> (x-y=w1267:u16)
        n704 = Select(t=w1243, s=w1260, f=w1242) -> (s? t:f=w1265:u16)
        n705 = Subtract(x=w1267, y=w1266) -> (x-y=w1245:u16)
        n706 = Subtract(x=w1265, y=w1245) -> (x-y=w1256:u16)
        n707 = Number To Boolean Array(number=w1245) -> (Boolean array=w1246:bool[])
        n708 = Or Array Elements(Boolean array=w1246) -> (logical OR=w1244:bool)
        n709 = Boolean To (0,1)(Boolean=w1244) -> (0, 1=w1251:i16)
        n710 = Boolean To (0,1)(Boolean="+ phase (APD 3 Gate)") -> (0, 1=w1254:i16)
        n711 = To Unsigned Byte Integer(number=w1251) -> (unsigned 8bit integer=w1248:u8)
        n712 = Multiply(x=w1254, y="Phase count adjustment (APD 3 Gate)") -> (x*y=w1252:i16)
        n713 = feedback #59(u8 0) -> (w1249:u8)
        n714 = Add(x=w1248, y=w1249) -> (x+y=w1247:u8)
        "APD 3 Gate Late Counter" <- w1247
        n715 = feedback-in #59(w1247) -> ()
        n716 = Add(x=w1256, y=w1252) -> (x+y=w1257:u16)
        n717 = feedback #60(i16 0) -> (w1259:i16)
        n718 = Subtract(x=w1259, y=w1252) -> (x-y=w1258:i16)
        "APD 3 Gate Relative Phase" <- w1258
        n719 = feedback-in #60(w1258) -> ()
        n720 = local read "APD Gate Operating Mode"() -> (w1241:u8)
        n721 = case shown="2" w1241 {
          tunnel: [TRUE FALSE w1275] -> w1261
          tunnel: w1263 -> [_ _ w1273]
          frame 0, Default {
          }
          frame 1 {
          }
          frame 2 {
            n722 = local read "Invert APD Gate"() -> (w1272:bool)
            n723 = Not(x=w1273) -> (.not. x?=w1274:bool)
            n724 = Select(t=w1274, s=w1272, f=w1273) -> (s? t:f=w1275:bool)
          }
        }
      }
    }
  }
  n725 = while "633 nm red  fluorescent laser interlacing (DO to IA 633 nm AOM ME amp)." {
    shift-right: [w1279] -> _
    shift-left: w2 -> [w1284]
    shift-right: [w1278] -> _
    shift-left: w3 -> [w1276]
    stop <- FALSE stop-if-true
    n726 = flat-sequence {
      tunnel: w1284 -> [w1287]
      tunnel: [w1288] -> w1282
      tunnel: [w1287] -> w1280
      tunnel: [w1286] -> w1277
      tunnel: w1276 -> [w1286]
      tunnel: [w1291] -> w1283
      tunnel: w1282 -> [w1291]
      tunnel: [w1290] -> w1281
      tunnel: w1280 -> [w1290]
      tunnel: w1277 -> [w1289]
      tunnel: [w1300] -> w1279
      tunnel: w1283 -> [w1320]
      tunnel: w1281 -> [w1317]
      tunnel: [w1309] -> w1278
      frame #0 {
        n727 = call "Loop Timer11"("Count(Ticks)"=w1287) -> ("Tick Count(Ticks)"=w1288:u16)
      }
      frame #1 {
        # "Then to PRL 440 amp"
        n728 = xnode "FPGA I/O Node"("Connector1/DIO32"=w1289) -> ()  [unwired: 1 in, 1 out]
      }
      frame #2 {
        n729 = feedback-in #61(w1320) -> ()
        n730 = feedback #61(w1320) -> (w1319:u16)
        n731 = Subtract(x=w1320, y=w1319) -> (x-y=w1318:u16)
        n732 = Subtract(x=w1318, y=w1317) -> (x-y=w1293:u16)
        n733 = Number To Boolean Array(number=w1293) -> (Boolean array=w1294:bool[])
        n734 = Or Array Elements(Boolean array=w1294) -> (logical OR=w1292:bool)
        n735 = Boolean To (0,1)(Boolean="+ phase (RI)") -> (0, 1=w1305:i16)
        n736 = Multiply(x=w1305, y="Phase count adjustment (RI)") -> (x*y=w1302:i16)
        n737 = Boolean To (0,1)(Boolean=w1292) -> (0, 1=w1299:i16)
        n738 = To Unsigned Byte Integer(number=w1299) -> (unsigned 8bit integer=w1296:u8)
        n739 = feedback #62(i16 0) -> (w1303:i16)
        n740 = feedback #63(u8 0) -> (w1297:u8)
        n741 = Add(x=w1296, y=w1297) -> (x+y=w1295:u8)
        "RI Late Counter" <- w1295
        n742 = feedback-in #63(w1295) -> ()
        n743 = Subtract(x=w1303, y=w1302) -> (x-y=w1301:i16)
        "RI Relative phase" <- w1301
        n744 = feedback-in #62(w1301) -> ()
        n745 = feedback #64(TRUE) -> (w1312:bool)
        n746 = case shown="2" "Red Laser Operating Mode" {
          tunnel: [TRUE FALSE w1326] -> w1309
          tunnel: w1312 -> [_ _ w1323]
          frame 0, Default {
          }
          frame 1 {
          }
          frame 2 {
            n747 = Not(x=w1323) -> (.not. x?=w1325:bool)
            n748 = Select(t=w1325, s="Invert RI", f=w1323) -> (s? t:f=w1326:bool)
          }
        }
        n749 = Not(x=w1312) -> (.not. x?=w1308:bool)
        n750 = Select(t="Red interlace ON count", s=w1308, f="Red interlace OFF count") -> (s? t:f=w1314:u16)
        n751 = Subtract(x=w1314, y=w1293) -> (x-y=w1306:u16)
        n752 = Add(x=w1306, y=w1302) -> (x+y=w1300:u16)
        n753 = feedback-in #64(w1308) -> ()
      }
    }
  }
  n754 = while "473 nm blue  fluorescent laser interlacing (DO to blue laser digital control input)." {
    shift-right: [w1330] -> _
    shift-left: w2 -> [w1335]
    shift-right: [w1329] -> _
    shift-left: w3 -> [w1327]
    stop <- FALSE stop-if-true
    n755 = flat-sequence {
      tunnel: w1335 -> [w1338]
      tunnel: [w1339] -> w1333
      tunnel: [w1338] -> w1331
      tunnel: [w1337] -> w1328
      tunnel: w1327 -> [w1337]
      tunnel: [w1342] -> w1334
      tunnel: w1333 -> [w1342]
      tunnel: [w1341] -> w1332
      tunnel: w1331 -> [w1341]
      tunnel: w1328 -> [w1340]
      tunnel: [w1351] -> w1330
      tunnel: w1334 -> [w1371]
      tunnel: w1332 -> [w1368]
      tunnel: [w1360] -> w1329
      frame #0 {
        n756 = call "Loop Timer14"("Count(Ticks)"=w1338) -> ("Tick Count(Ticks)"=w1339:u16)
      }
      frame #1 {
        n757 = xnode "FPGA I/O Node"("Connector1/DIO28"=w1340) -> ()  [unwired: 1 in, 1 out]
      }
      frame #2 {
        n758 = feedback-in #65(w1371) -> ()
        n759 = feedback #65(w1371) -> (w1370:u16)
        n760 = Subtract(x=w1371, y=w1370) -> (x-y=w1369:u16)
        n761 = Subtract(x=w1369, y=w1368) -> (x-y=w1344:u16)
        n762 = Number To Boolean Array(number=w1344) -> (Boolean array=w1345:bool[])
        n763 = Or Array Elements(Boolean array=w1345) -> (logical OR=w1343:bool)
        n764 = Boolean To (0,1)(Boolean="+ phase (BI D)") -> (0, 1=w1356:i16)
        n765 = Multiply(x=w1356, y="Phase count adjustment (BI D)") -> (x*y=w1353:i16)
        n766 = Boolean To (0,1)(Boolean=w1343) -> (0, 1=w1350:i16)
        n767 = To Unsigned Byte Integer(number=w1350) -> (unsigned 8bit integer=w1347:u8)
        n768 = feedback #66(i16 0) -> (w1354:i16)
        n769 = feedback #67(u8 0) -> (w1348:u8)
        n770 = Add(x=w1347, y=w1348) -> (x+y=w1346:u8)
        "Blue Late Counter (D)" <- w1346
        n771 = feedback-in #67(w1346) -> ()
        n772 = Subtract(x=w1354, y=w1353) -> (x-y=w1352:i16)
        "BI Relative phase (D)" <- w1352
        n773 = feedback-in #66(w1352) -> ()
        n774 = feedback #68(TRUE) -> (w1363:bool)
        n775 = case shown="2" "Blue Laser Operating Mode (D)" {
          tunnel: [TRUE FALSE w1377] -> w1360
          tunnel: w1363 -> [_ _ w1374]
          frame 0, Default {
          }
          frame 1 {
          }
          frame 2 {
            n776 = Not(x=w1374) -> (.not. x?=w1376:bool)
            n777 = Select(t=w1376, s="Invert BI (D)", f=w1374) -> (s? t:f=w1377:bool)
          }
        }
        n778 = Not(x=w1363) -> (.not. x?=w1359:bool)
        n779 = Select(t="Blue interlace ON count (D)", s=w1359, f="Blue interlace OFF count (D)") -> (s? t:f=w1365:u16)
        n780 = Subtract(x=w1365, y=w1344) -> (x-y=w1357:u16)
        n781 = Add(x=w1357, y=w1353) -> (x+y=w1351:u16)
        n782 = feedback-in #68(w1359) -> ()
      }
    }
  }
  n783 = while "Blue fluorescent laser interlacing (AO control direct to laser)." {
    shift-right: [w1383] -> _
    shift-left: w2 -> [w1386]
    shift-right: [w1380] -> _
    shift-left: i16 0 -> [w1378]
    stop <- FALSE stop-if-true
    n784 = flat-sequence {
      tunnel: w1386 -> [w1389]
      tunnel: [w1390] -> w1385
      tunnel: [w1389] -> w1384
      tunnel: [w1388] -> w1379
      tunnel: w1378 -> [w1388]
      tunnel: [w1393] -> w1382
      tunnel: w1385 -> [w1393]
      tunnel: [w1392] -> w1381
      tunnel: w1384 -> [w1392]
      tunnel: w1379 -> [w1391]
      tunnel: [w1403] -> w1383
      tunnel: [w1419] -> w1380
      tunnel: w1382 -> [w1431]
      tunnel: w1381 -> [w1428]
      frame #0 {
        n785 = call "Loop Timer13"("Count(Ticks)"=w1389) -> ("Tick Count(Ticks)"=w1390:u16)
      }
      frame #1 {
        n786 = xnode "FPGA I/O Node"("Connector0/AO3"=w1391) -> ()  [unwired: 1 in, 1 out]
      }
      frame #2 {
        n787 = Subtract(x="Blue OFF count (AO)", y="Blue current ON count adj (AO)") -> (x-y=w1412:u16)
        n788 = feedback-in #69(w1431) -> ()
        n789 = feedback #69(w1431) -> (w1430:u16)
        n790 = Add(x="Blue current ON count adj (AO)", y="Blue ON count (AO)") -> (x+y=w1413:u16)
        n791 = Subtract(x=w1431, y=w1430) -> (x-y=w1429:u16)
        n792 = Subtract(x=w1429, y=w1428) -> (x-y=w1396:u16)
        n793 = Number To Boolean Array(number=w1396) -> (Boolean array=w1397:bool[])
        n794 = Boolean To (0,1)(Boolean="+ phase (BI AO)") -> (0, 1=w1409:i16)
        n795 = Or Array Elements(Boolean array=w1397) -> (logical OR=w1395:bool)
        n796 = Boolean To (0,1)(Boolean=w1395) -> (0, 1=w1402:i16)
        n797 = Multiply(x=w1409, y="Phase count adjustment (BI AO)") -> (x*y=w1405:i16)
        n798 = To Unsigned Byte Integer(number=w1402) -> (unsigned 8bit integer=w1398:u8)
        n799 = feedback #70(u8 0) -> (w1400:u8)
        n800 = Add(x=w1398, y=w1400) -> (x+y=w1399:u8)
        "BI Late Counter (AO)" <- w1399
        n801 = feedback-in #70(w1399) -> ()
        n802 = feedback #71(i16 0) -> (w1406:i16)
        n803 = Subtract(x=w1406, y=w1405) -> (x-y=w1404:i16)
        "BI Relative phase (AO)" <- w1404
        n804 = feedback-in #71(w1404) -> ()
        n805 = feedback #72(TRUE) -> (w1423:bool)
        n806 = case shown="2" "BI Operating Mode (AO)" {
          tunnel: [TRUE FALSE w1447] -> w1414
          tunnel: w1423 -> [_ _ w1444]
          frame 0, Default {
          }
          frame 1 {
          }
          frame 2 {
            n807 = Not(x=w1444) -> (.not. x?=w1446:bool)
            n808 = Select(t=w1446, s="Invert BI (AO)", f=w1444) -> (s? t:f=w1447:bool)
          }
        }
        n809 = And(x=w1414, y="Blue FB On/Off") -> (x .and. y?=w1415:bool)
        n810 = case shown="True" w1415 {
          tunnel: "BI Current Out" -> [w1432 _]
          tunnel: [w1432 w1434] -> w1418
          frame False {
          }
          frame True {
            n811 = local read "Blue Intensity"() -> (w1433:i16)
            n812 = Bundle("P5"="P5", "I5"="I5", "D5"="D5") -> (w1435:cluster{"P5":i16, "I5":i16, "D5":i16})  [unwired: 1 in]
            n813 = call "Slower PID.vi"("process variable"=w1433, "reset?"="Blue FB Reset", "setpoint"="Blue FB Setpoint", "PID gains (x 2^8)"=w1435, "output range"=cluster{"output high":i16, "output low":i16} {"output high"=32767, "output low"=0} ("Green FB output range")) -> ("output"=w1434:i16)  [unwired: 10 out]
          }
        }
        n814 = Not(x=w1423) -> (.not. x?=w1420:bool)
        n815 = Select(t=w1413, s=w1420, f=w1412) -> (s? t:f=w1425:u16)
        n816 = Subtract(x=w1425, y=w1396) -> (x-y=w1407:u16)
        n817 = Add(x=w1407, y=w1405) -> (x+y=w1403:u16)
        n818 = feedback-in #72(w1420) -> ()
        n819 = Boolean To (0,1)(Boolean=w1414) -> (0, 1=w1394:i16)
        n820 = Multiply(x=w1394, y=w1418) -> (x*y=w1419:i16)
      }
    }
  }
